vi "Measurement.vi"(0 "Position":T7(array[cluster]) {"Z" format="%.1f"; "Y" format="%.1f"; "X" format="%.1f"}, 1 "setup":T8=enum."Show Setup", 2 "Post Process":T5, 4 "File":T9, 5 "Results file":path, 7 "Raw data file":path, 11 "Setup filename":string) -> (14 "2nd plot":cluster{"Xo":dbl, "Delta X":dbl, dbl[]}[](graph), 19 "Status Out":T4)   [LabVIEW 2010]
uses:
  Anemometry Sub Vis/Controls/Save_Data.ctl
  Anemometry Sub Vis/Controls/Setup.ctl
  Anemometry Sub Vis/Controls/Graph_Type.ctl
  Anemometry Sub Vis/Controls/Post_Process.ctl
  Anemometry Sub Vis/Gen Trav/Multi_Run_Status.ctl
  Anemometry Sub Vis/Controls/Board_Types.ctl
  Anemometry Sub Vis/File/Setup_Filetype.ctl
  Anemometry Sub Vis/Controls/Block_start_and_end.ctl
  ADAM Client/Sub VIs/ADAM Controls/Traverse_Level_State.ctl
  Anemometry Sub Vis/Globals/Trav_pos_global.vi
  Anemometry Sub Vis/Globals/Meas_global.vi
  Anemometry Sub Vis/Acquisition/Data_Translation/DataTranslation_global.vi
  Anemometry Sub Vis/Acquisition/PWA/PWAtasksGLOBAL.vi
  Anemometry Sub Vis/Globals/Preference_global.vi
  Anemometry Sub Vis/Globals/LDA_meas_global_1.vi
  Anemometry Sub Vis/Globals/Dynamic_call_global.ph.vi
  Anemometry Sub Vis/Globals/LDA_meas_global_2.vi
  Anemometry Sub Vis/Globals/Plug_in_data_global.vi
panel:
  in  "PP next block":bool
  out "Pause message":string
  out "Statistics":string[][](table)
  in  "Tab Control":T1(tab)
  out "Measurement time (min)":dbl=6.0 format="%.2f"
  in  "No of bins":i32=80
  in  "Show Smoth":bool=TRUE
  in  "Second Graph":T3={"Plot 1"=2, "Plot 2"=1, "Save graph"=0, "Plot Type"=enum."Vel histogram"} {"Save graph" items=["Do not save plot", "Save plot"]; "Plot 2" items=["Nothing", "LDA (U)", "LDA (W)", "HW (HW) LDA Sync", "HW (HW)", "RV (WT)"]; "Plot 1" items=["Nothing", "LDA (U)", "LDA (W)", "HW (HW) LDA Sync", "HW (HW)", "RV (WT)"]}
  in  "First Graph":T3={"Plot 1"=1, "Plot 2"=2, "Save graph"=0, "Plot Type"=enum."Velocity trace"} {"Save graph" items=["Do not save plot", "Save plot"]; "Plot 2" items=["Nothing", "LDA (U)", "LDA (W)", "HW (HW) LDA Sync", "HW (HW)", "RV (WT)"]; "Plot 1" items=["Nothing", "LDA (U)", "LDA (W)", "HW (HW) LDA Sync", "HW (HW)", "RV (WT)"]}
  out "First plot":cluster{"Xo":dbl, "Delta X":dbl, dbl[]}[](graph)
  in  "Comments":string
  out "BSA Diagnostic info":string[][](table)
  out "uv":dbl[][](graph)=[[-0.041806189081711534, -0.046435429052714985, -0.04035660097427599, -0.042187605126076694, -0.042052555599004206]]
  out "u^4":dbl[][](graph)
  out "u^3":dbl[][](graph)
  out "u^2":dbl[][](graph)=[[0.09743628875280319, 0.10575821456272283, 0.10126262927293661, 0.09890442087602569, 0.1022948212436432]]
  out "U":dbl[][](graph)=[[0.8295029456391334, 0.8915896983798417, 0.8415763502225625, 0.8394746126219594, 0.8466062785395404]]
  in  "Block average display control":cluster{"Name":string, "Include":bool}[](array[cluster])=[{"Name"="FF (C)", "Include"=FALSE}]
  out "Array U":dbl[][](array[numeric]) format="%.2e"
  out "Array u^2":dbl[][](array[numeric]) format="%.2e"
  out "Actual Sampling freq":dbl=100.0 format="%.1f"
  in  "Desired Sampling freq (Hz)":dbl=100.0 format="%.1f"
  in  "Correlate?":T6(ring)
  out "Current Block No":i32=5
  in  "Pause":bool
  in  "No of Blocks":i32=5
  in  "stop":bool
  in  "No of samples":i32=1000 min=0 step=1
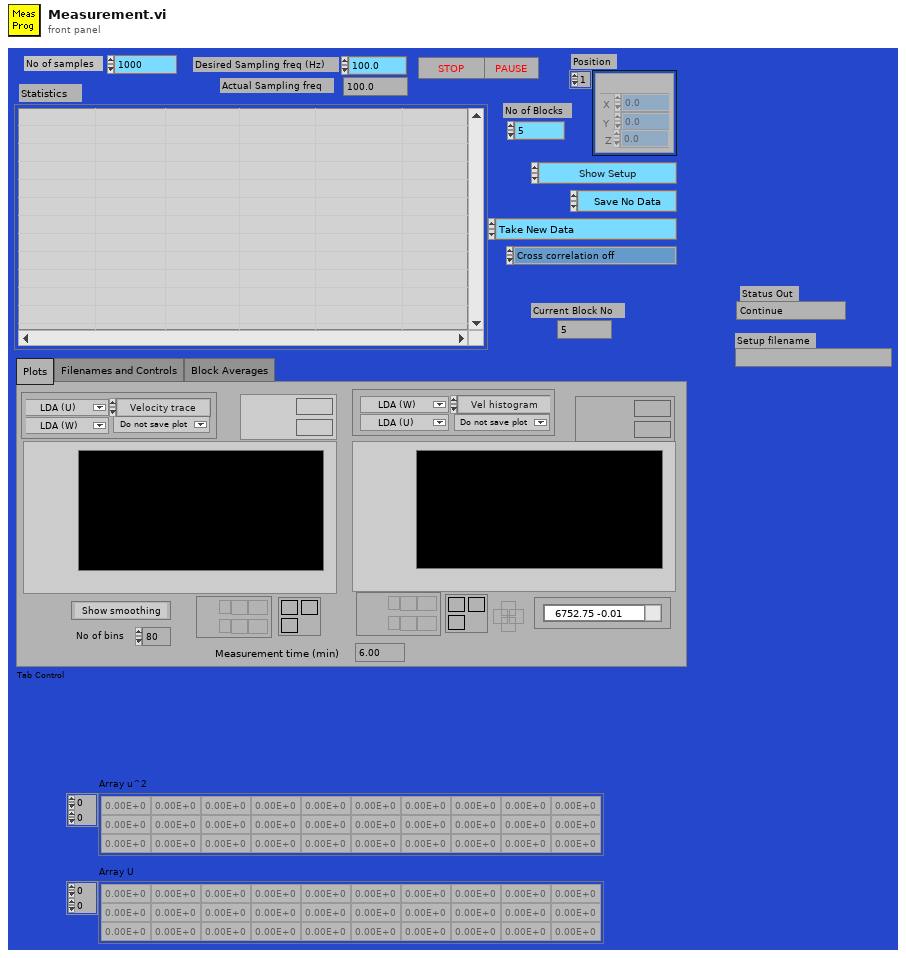
[diagram p1: front panel]
types:
  T1 = enum32{"Plots", "Filenames and Controls", "Block Averages"}
  T2 = typedef "Graph_Type.ctl" = enum16{"Show no graph", "Voltage trace", "Velocity trace", "Vel histogram", "Spectrum", "f.E(f) v Log f", "Auto-Corr"}
  T3 = cluster{"Plot 1":u16, "Plot 2":u16, "Save graph":u16, "Plot Type":T2}
  T4 = typedef "Multi_Run_Status.ctl" = enum16{"Continue", "Jump to Next Point", "Jump to Next Row", "Jump To Fall Back", "Terminate Run"}
  T5 = typedef "Post_Process.ctl" = enum16{"Take New Data", "Post Process Raw Data File"}
  T6 = enum16{"Cross correlation off", "Show correlation panel", "Correlate without activating panel"}
  T7 = cluster{"Name":string, "X":dbl, "Y":dbl, "Z":dbl}[]
  T8 = typedef "Setup.ctl" = enum16{"Run Program", "Show Setup", "Save Current Setup", "Setup Front Panel"}
  T9 = typedef "Save_Data.ctl" = enum16{"Save No Data", "Save Data"}
  T10 = enum32{"Bad", "Idle", "Run top level", "Running"}
  T11 = enum16{"Velocity", "Transit time", "Arrival time"}
  T12 = enum16{"Save no data", "Save data in new files", "Save data in existing files"}
  T13 = typedef "Board_Types.ctl" = enum16{"Simulate", "Local ADAM", "Server ADAM", "NI-DAQmx", "NI-DAQmxBase", "ADC488", "DT LV-link"}
  T14 = typedef "Setup_Filetype.ctl" = enum16{"Measurement Setups", "Calibration Setups", "General", "Results File Plotter Setups", "Speed Calib Tweaks"}
  T15 = typedef "Block_start_and_end.ctl" = cluster{"Started":dbl, "Ended":dbl, "Analogue Frequency Hz":dbl}
  T16 = typedef "Traverse_Level_State.ctl" = enum16{"Running", "Complete"}
  T17 = typedef "Traverse_cluster.ctl" = cluster{"Start X":dbl, "Start Y":dbl, "Start Z":dbl, "End X":dbl, "End Y":dbl, "End Z":dbl, "No. of pts.":i32, "Spacing":T18, "Filename":path, "Tunnel Speed":dbl, "Averaging time (min)":dbl, "Extra Commands":string, "Specific Arguments":string, "Emission Rate (l/min)":dbl, "Trace Gas Concentration (%)":dbl, "Density Ratio":string, "Comments":string, "Row No":i32, "Row Type Selector":T19, "Completion time":string, "Row Duration (mins)":dbl, "No. of Valid pts.":i32, "Meas Setup File":string}
  T18 = typedef "Spacing.ctl" = enum16{"Linear", "Log", "Gauss", "Specified", "N/A"}
  T19 = typedef "Multi_run_mode.ctl" = enum16{"Move Traverse Only", "Set Tunnel Speed Only", "Set Source Only", "Set Measurement Conditions", "Single Measurement", "Vertical Profile", "Lateral Profile", "Longitudinal Profile", "Explore Volume", "Multi-Axis Profile", "Auto Calibrate", "Meas Fast FID Bkgnd", "Check Beam Power", "Scanning Valve Measurement", "Run VI Named:", "Set ADAM Ch", "Wait (minutes)", "Send Message", "Synchronize With:", "Fall Back to this Row", "Turn Off Row Repeating", "Blank Row"}
  T20 = typedef "Analysis_info_cluster.ctl" = cluster{"Colour":u32, "Inst type":T21, "Inst name":string, "Symbol":string, "Code name":string, "Extra Info":string, "Inst Array":T22, "Index":i32, "Voltage Index":i32, "Extra Titles":string[], "Extra Values":string[]}
  T21 = typedef "Inst_type.ctl" = enum16{"Propeller anemometer", "Raw voltage", "Pressure Transducer", "Pitot-static tube", "Preston tube", "Hot wire", "Cross wire 1", "Cross wire 2", "Generic Linear", "Generic Polynomial", "Generic BackPoly", "Fast FID", "Thermocouple", "Cold wire", "Pulsed Wire", "LDA Vel", "LDA Tran time", "LDA Arr time"}
  T22 = typedef "Instrument_Array.ctl" = enum16{"PWA", "LDA", "Analogue"}
  T23 = enum16{"Velocity", "Transit time", "Arrival time"}[]
  T24 = typedef "BSA_Type.ctl" = enum16{"57N11", "BSA F60"}
  T25 = typedef "BSA_info_Cluster.ctl" = cluster{"GPIB Address":string, "No of Check Bytes":i32, "Extra Info":string, "COLOUR":u32, "Wavelength (nm)":dbl}
  T26 = typedef "Ch_and_Spans.ctl" = cluster{"high limit (10V)":sgl, "low limit (-10V)":sgl, "Ch No":i16, "Var name":string, "Use Latest Calib":bool}
  T27 = typedef "Velocity_cluster.ctl" = cluster{"Name":string, "U":dbl, "u^2":dbl, "u^3/(u^2)^(1.5)":dbl, "u^4/(u^2)^2 -3":dbl, "% u'/U":dbl, "Mean % Err":dbl, "u^4":dbl}
  T28 = typedef "Analysis_type_cluster.ctl" = cluster{"Analysis type":T29, "Indicies":i32[], "Name":string, "Inst Array":T22, "Info index":i32}
  T29 = typedef "Analysis_type_Enum.ctl" = enum16{"Slow Response", "Fast Response", "Weighted Fast Response", "Fast FID", "Weighted Fast FID", "Cross Wire", "Weighted Cross Wire", "Weighted LDA"}
  T30 = cluster{"Insts for plotting[0]":u16, "Insts for plotting[1]":u16}
  T31 = typedef "PWA_Data.ctl" = enum16{"No PWA Data", "One Ch PWA"}
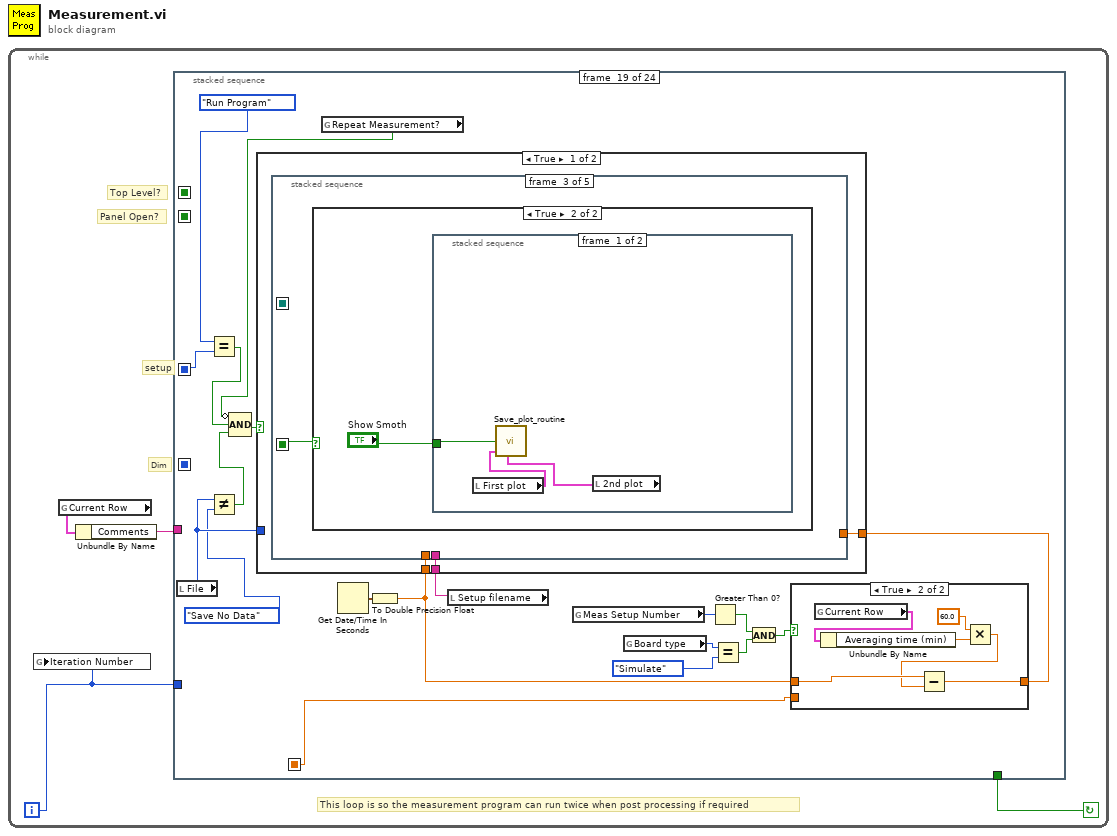
[diagram p0: block diagram]
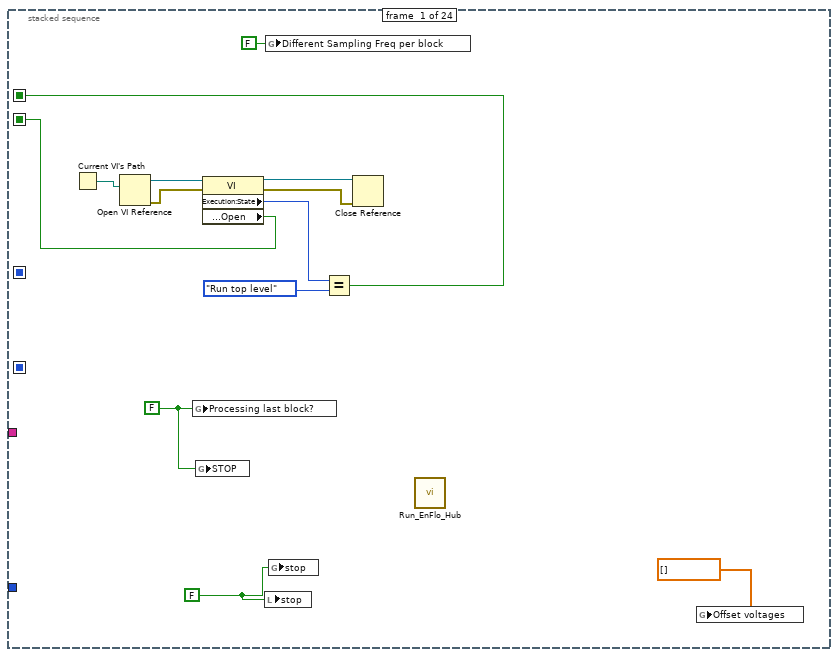
[diagram p2: hidden frame]
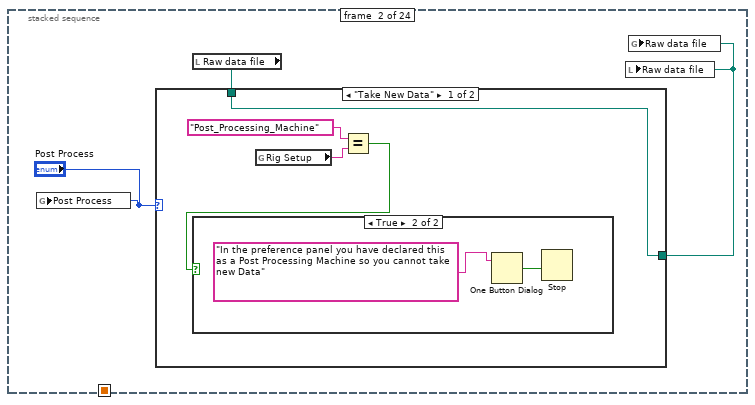
[diagram p3: hidden frame]
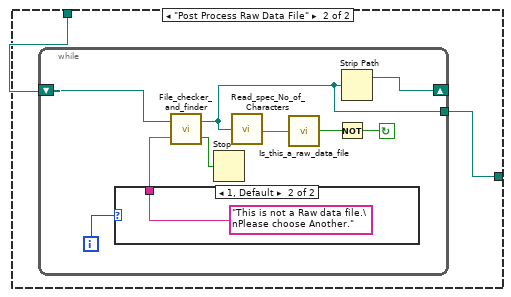
[diagram p5: hidden frame]
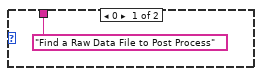
[diagram p6: hidden frame]
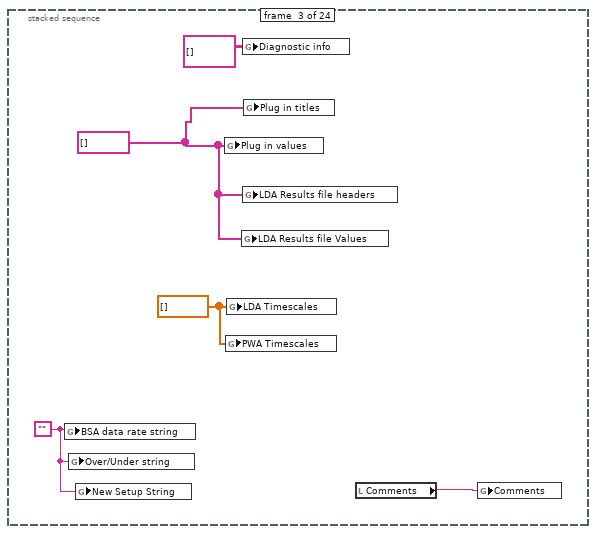
[diagram p7: hidden frame]
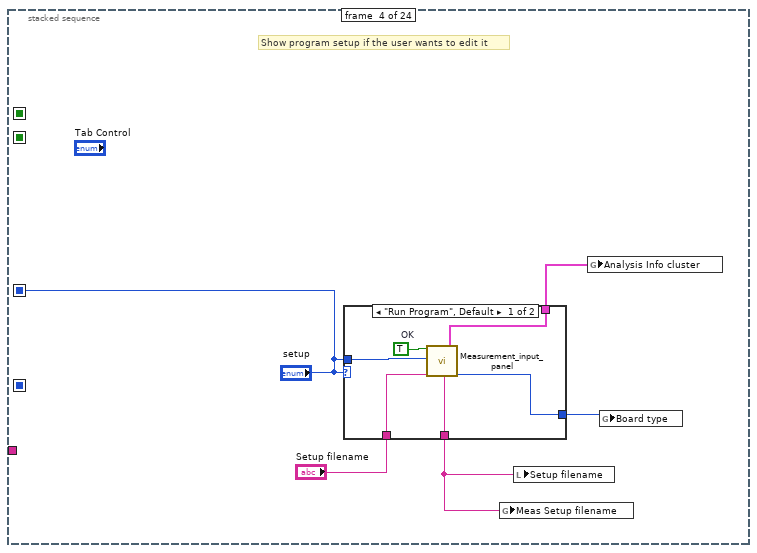
[diagram p8: hidden frame]
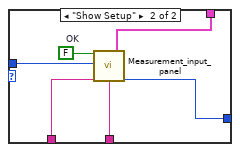
[diagram p9: hidden frame]
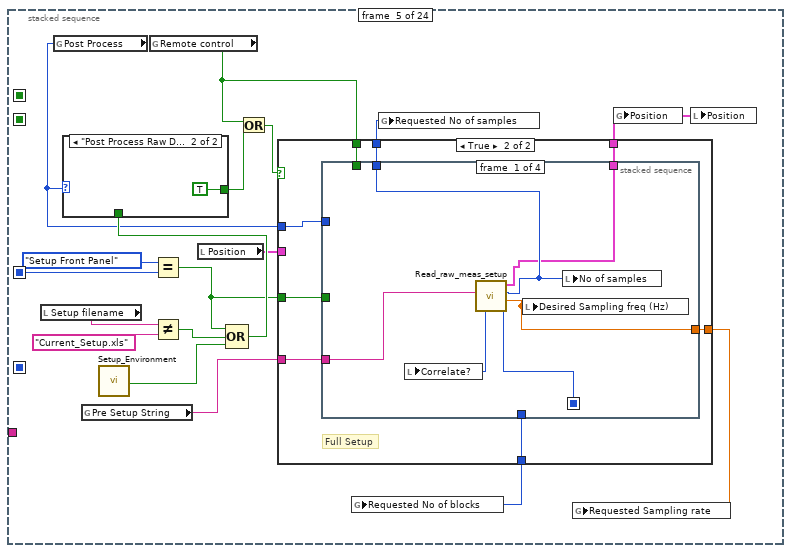
[diagram p10: hidden frame]
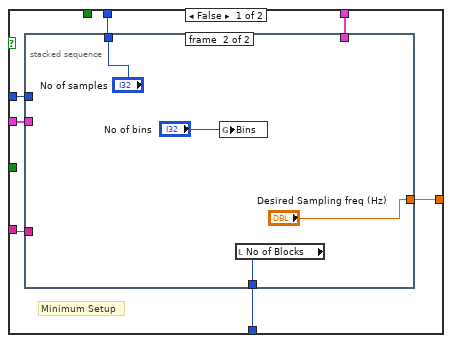
[diagram p12: hidden frame]
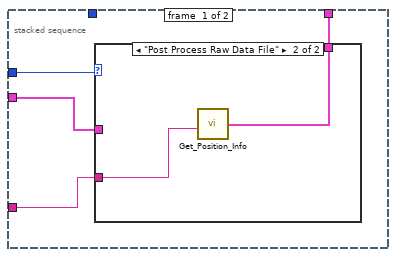
[diagram p13: hidden frame]
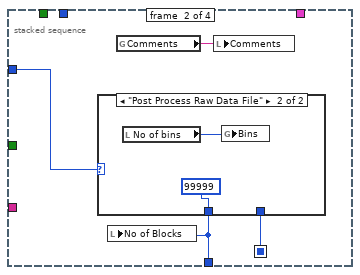
[diagram p15: hidden frame]
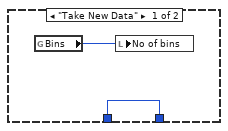
[diagram p16: hidden frame]
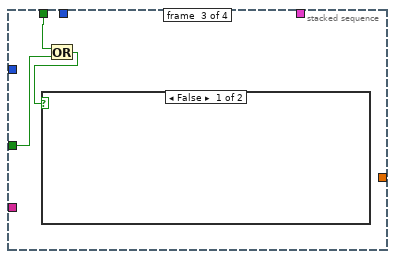
[diagram p17: hidden frame]
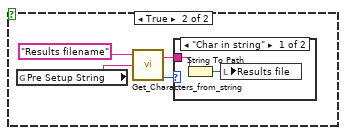
[diagram p18: hidden frame]
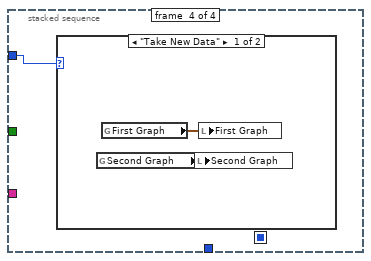
[diagram p20: hidden frame]
diagram:
  n1 = while {
    i -> [w1]
    stop <- w2 continue-if-true
    # "This loop is so the measurement program can run twice when post processing if required"
    # "Panel Open?"
    # "Top Level?"
    # "setup"
    # "Dim"
    n2 = global write "Meas_global.vi" "Iteration Number"(w1) -> ()
    n3 = global read "Trav_pos_global.vi" "Current Row"() -> (w3:T17)
    n4 = Unbundle By Name(w3) -> ("Comments"=w4:string)
    n5 = stacked-sequence {
      seq-local: [_ _ _ _ _ _ _ _ w187 _ _ _ _ _ _ _ _ _ _ _ _ _ _ _] -> [_ _ _ _ _ _ _ _ _ _ _ _ _ _ _ _ _ w625 _ _ _ _ _ _]
      seq-local: [_ _ _ "setup" _ _ _ _ _ _ _ _ _ _ _ _ _ _ _ _ _ _ _ _] -> [_ _ _ _ w71 _ _ _ w179 w264 _ _ _ _ w525 w563 w570 w626 w934 w1010 w1038 _ _ w1115]
      seq-local: [_ _ _ _ _ _ _ _ _ _ _ _ _ _ _ _ w566 _ _ _ _ _ _ _] -> [_ _ _ _ _ _ _ _ _ _ _ _ _ _ _ _ _ w624 w917 _ _ _ _ _]
      seq-local: [w7 _ _ _ _ _ _ _ _ _ _ _ _ _ _ _ _ _ _ _ _ _ _ _] -> [_ _ _ _ _ _ _ _ _ w244 _ _ _ _ w521 _ _ w623 _ _ _ _ _ _]
      seq-local: [w6 _ _ _ _ _ _ _ _ _ _ _ _ _ _ _ _ _ _ _ _ _ _ _] -> [_ _ _ _ _ _ _ _ _ _ _ _ w364 _ _ _ _ _ _ _ _ _ _ _]
      tunnel: w4 -> [_ _ _ _ _ _ _ w172 _ _ _ _ _ _ _ _ _ _ _ _ _ _ w1081 _]
      tunnel: w1 -> [_ _ _ _ _ _ _ _ _ _ _ _ _ _ _ _ _ _ _ _ _ _ w1076 _]
      tunnel: [_ _ _ _ _ _ _ _ _ _ _ _ _ _ _ _ _ _ _ _ _ _ w1075 _] -> w2
      frame #0 {
        w15 = FALSE ("Processing last block?")
        w16 = FALSE ("stop")
        n6 = Current VI's Path() -> (path=w8:path)
        n7 = Open VI Reference(vi path=w8) -> (vi reference=w9:refnum<vi>, error out=w10:errorcluster)  [unwired: 1 in, 4 out]
        n8 = global write "Meas_global.vi" "Processing last block?"(w15) -> ()
        n9 = global write "PWAtasksGLOBAL.vi" "STOP"(w15) -> ()
        n10 = property class="VI"(reference=w9, error in=w10) -> (reference out=w11:refnum<vi>, error out=w12:errorcluster, "Execution:State"=w13:T10, "Front Panel.Open"=w6:bool)
        n11 = local write "stop"(w16) -> ()
        n12 = global write "DataTranslation_global.vi" "Different Sampling Freq per block"(FALSE ("Different Sampling Freq per block")) -> ()
        n13 = global write "Meas_global.vi" "stop"(w16) -> ()
        n14 = Equal?(x=w13, y=T10."Run top level" ("Exec.State")) -> (x = y?=w7:bool)
        n15 = Close Reference(reference=w11, error in (no error)=w12) -> ()  [unwired: 1 out]
        n16 = call "Run_EnFlo_Hub.vi"() -> ()  [unwired: 8 out]
        n17 = global write "Meas_global.vi" "Offset voltages"(dbl[] [] ("Offset voltages used")) -> ()
      }
      frame #1 {
        n18 = global write "Meas_global.vi" "Post Process"("Post Process") -> ()
        n19 = local read "Raw data file"() -> (w20:path)
        n20 = case shown="\"Take New Data\"" "Post Process" {
          tunnel: [w24 w28] -> w19
          tunnel: w20 -> [w24 w27]
          frame "Take New Data" {
            n21 = global read "Preference_global.vi" "Rig Setup"() -> (w23:string)
            n22 = Equal?(x="Post_Processing_Machine" ("Rig Setup"), y=w23) -> (x = y?=w21:bool)
            n23 = case shown="True" w21 {
              frame False {
              }
              frame True {
                n24 = One Button Dialog(message="In the preference panel you have declared this as a Post Processing Machine so you cannot take new Data") -> (true=w25:bool)  [unwired: 1 in]
                n25 = Stop(stop? (T)=w25) -> ()
              }
            }
          }
          frame "Post Process Raw Data File" {
            n26 = while {
              tunnel: [w30] -> w28
              shift-left: w27 -> [w32]
              shift-right: [w31] -> _
              i -> [w33]
              stop <- w34 continue-if-true
              n27 = case shown="1, Default" w33 {
                tunnel: ["Find a Raw Data File to Post Process" ("Promp if not found") "This is not a Raw data file.\nPlease choose Another." ("Promp if not found")] -> w37
                frame 0 {
                }
                frame 1, Default {
                }
              }
              n28 = call "File_checker_and_finder.vi"("Promp if not found"=w37, "Filename In"=w32) -> ("cancelled"=w29:bool, "Filename Out"=w30:path)
              n29 = Stop(stop? (T)=w29) -> ()
              n30 = call "Read_spec_No_of_Characters.vi"("Filename"=w30) -> ("character string"=w36:string)  [unwired: 1 out]
              n31 = call "Is_this_a_raw_data_file.vi"("character string"=w36) -> ("Raw Dat File?"=w35:bool)  [unwired: 2 out]
              n32 = Not(x=w35) -> (.not. x?=w34:bool)
              n33 = Strip Path(path=w30) -> (stripped path=w31:path)  [unwired: 1 out]
            }
          }
        }
        n34 = local write "Raw data file"(w19) -> ()
        n35 = global write "Meas_global.vi" "Raw data file"(w19) -> ()
      }
      frame #2 {
        w42 = dbl[] [] ("LDA Timescales")
        w41 = string[] [] ("Plug in values")
        w44 = ""
        n36 = global write "Meas_global.vi" "BSA data rate string"(w44) -> ()
        n37 = global write "Meas_global.vi" "Over/Under string"(w44) -> ()
        n38 = global write "Meas_global.vi" "New Setup String"(w44) -> ()
        n39 = global write "Dynamic_call_global.ph.vi" "Plug in values"(w41) -> ()
        n40 = global write "PWAtasksGLOBAL.vi" "PWA Timescales"(w42) -> ()
        n41 = global write "LDA_meas_global_1.vi" "LDA Timescales"(w42) -> ()
        n42 = global write "LDA_meas_global_1.vi" "LDA Results file Values"(w41) -> ()
        n43 = global write "Meas_global.vi" "Diagnostic info"(string[][] [] ("Diagnostic info")) -> ()
        n44 = global write "LDA_meas_global_1.vi" "LDA Results file headers"(w41) -> ()
        n45 = global write "Dynamic_call_global.ph.vi" "Plug in titles"(w41) -> ()
        n46 = local read "Comments"() -> (w43:string)
        n47 = global write "Meas_global.vi" "Comments"(w43) -> ()
      }
      frame #3 {
        # "Show program setup if the user wants to edit it"
        n48 = case shown="\"Run Program\", Default" "setup" {
          tunnel: [w54 w60] -> w49
          tunnel: [w53 w59] -> w48
          tunnel: "Setup filename" -> [w52 w58]
          tunnel: [w51 w57] -> w45
          tunnel: "setup" -> [w50 w56]
          frame "Run Program", Default {
            w55 = TRUE  # OK
            n49 = call "Measurement_input_panel.vi"("OK"=w55, "setup"=w50, "Setup filename"=w52) -> ("Setup filename out"=w51:string, "Analysis Info cluster"=w54:T20[], "Board type"=w53:T13)  [unwired: 14 out]
          }
          frame "Show Setup" {
            w61 = FALSE  # OK
            n50 = call "Measurement_input_panel.vi"("OK"=w61, "setup"=w56, "Setup filename"=w58) -> ("Setup filename out"=w57:string, "Analysis Info cluster"=w60:T20[], "Board type"=w59:T13)  [unwired: 14 out]
          }
        }
        n51 = global write "Meas_global.vi" "Meas Setup filename"(w45) -> ()
        n52 = local write "Setup filename"(w45) -> ()
        n53 = global write "Meas_global.vi" "Analysis Info cluster"(w49) -> ()
        n54 = global write "Meas_global.vi" "Board type"(w48) -> ()
      }
      frame #4 {
        n55 = local read "Setup filename"() -> (w75:string)
        n56 = global read "Meas_global.vi" "Post Process"() -> (w70:T5)
        n57 = global read "Meas_global.vi" "Pre Setup String"() -> (w66:string)
        n58 = call "Setup_Environment.vi"() -> ("First Time"=w67:bool)  [unwired: 1 in]
        n59 = global read "Meas_global.vi" "Remote control"() -> (w63:bool)
        n60 = Equal?(x=Setup."Setup Front Panel" ("setup"), y=w71) -> (x = y?=w62:bool)
        n61 = Not Equal?(x=w75, y="Current_Setup.xls" ("Setup filename")) -> (x != y?=w73:bool)
        n62 = local read "Position"() -> (w64:T7)
        n63 = Compound Arithmetic op=OR(w62, w73, w67) -> (w72:bool)
        n64 = case shown="\"Post Process Raw Data File\"" w70 {
          tunnel: [w80 TRUE] -> w79
          tunnel: w72 -> [w80 _]
          frame "Take New Data" {
          }
          frame "Post Process Raw Data File" {
          }
        }
        n65 = Or(x=w63, y=w79) -> (x .or. y?=w78:bool)
        n66 = case shown="True" w78 {
          tunnel: w70 -> [w84 w107]
          tunnel: [w88 w106] -> w68
          tunnel: [w87 w101] -> w77
          tunnel: [w86 w105] -> w76
          tunnel: [w85 w104] -> w65
          tunnel: w66 -> [w83 w103]
          tunnel: w64 -> [w82 _]
          tunnel: w63 -> [_ w102]
          tunnel: w62 -> [_ w100]
          frame False {
            # "Minimum Setup"
            n67 = stacked-sequence {
              tunnel: [_ "Desired Sampling freq (Hz)"] -> w88
              tunnel: [_ w98] -> w87
              tunnel: [_ "No of samples"] -> w86
              tunnel: [w91 _] -> w85
              tunnel: w84 -> [w92 _]
              tunnel: w83 -> [w90 _]
              tunnel: w82 -> [w89 _]
              frame #0 {
                n68 = case shown="\"Post Process Raw Data File\"" w92 {
                  tunnel: [w93 w94] -> w91
                  tunnel: w89 -> [w93 _]
                  tunnel: w90 -> [_ w95]
                  frame "Take New Data" {
                  }
                  frame "Post Process Raw Data File" {
                    n69 = call "Get_Position_Info.vi"("Input string"=w95) -> ("Position"=w94:T7)
                  }
                }
              }
              frame #1 {
                n70 = global write "Meas_global.vi" "Bins"("No of bins") -> ()
                n71 = local read "No of Blocks"() -> (w98:i32)
              }
            }
          }
          frame True {
            # "Full Setup"
            n72 = stacked-sequence {
              seq-local: [w110 _ _ _] -> [_ w115 _ _]
              tunnel: w107 -> [_ w116 _ w131]
              tunnel: [w113 _ _ _] -> w106
              tunnel: [w112 _ _ _] -> w105
              tunnel: [w108 _ _ _] -> w104
              tunnel: w103 -> [w111 _ _ _]
              tunnel: w102 -> [_ _ w124 _]
              tunnel: [_ w114 _ _] -> w101
              tunnel: w100 -> [_ _ w123 _]
              frame #0 {
                n73 = call "Read_raw_meas_setup.vi"("Setup file string"=w111) -> ("No of Blocks"=w110:i32, "Sampling freq (Hz)"=w113:dbl, "No of samples"=w112:i32, "Position"=w108:T7, "Correlate?"=w109:T6)  [unwired: 4 out]
                n74 = local write "Correlate?"(w109) -> ()
                n75 = local write "Desired Sampling freq (Hz)"(w113) -> ()
                n76 = local write "No of samples"(w112) -> ()
              }
              frame #1 {
                n77 = case shown="\"Post Process Raw Data File\"" w116 {
                  tunnel: [w119 99999 ("No of Blocks")] -> w114
                  tunnel: w115 -> [w119 _]
                  frame "Take New Data" {
                    n78 = global read "Meas_global.vi" "Bins"() -> (w118:i32)
                    n79 = local write "No of bins"(w118) -> ()
                  }
                  frame "Post Process Raw Data File" {
                    n80 = local read "No of bins"() -> (w120:i32)
                    n81 = global write "Meas_global.vi" "Bins"(w120) -> ()
                  }
                }
                n82 = local write "No of Blocks"(w114) -> ()
                n83 = global read "Meas_global.vi" "Comments"() -> (w117:string)
                n84 = local write "Comments"(w117) -> ()
              }
              frame #2 {
                n85 = Or(x=w124, y=w123) -> (x .or. y?=w122:bool)
                n86 = case shown="False" w122 {
                  frame False {
                  }
                  frame True {
                    n87 = global read "Meas_global.vi" "Pre Setup String"() -> (w125:string)
                    n88 = call "Get_Characters_from_string.vi"("Input string"=w125, "Variable name"="Results filename") -> ("Status"=w128:enum16{"Char in string", "Char not in string"}, "Value"=w127:string)  [unwired: 1 in]
                    n89 = case shown="\"Char in string\"" w128 {
                      tunnel: w127 -> [w130 _]
                      frame "Char in string" {
                        n90 = String To Path(string=w130) -> (path=w129:path)
                        n91 = local write "Results file"(w129) -> ()
                      }
                      frame "Char not in string" {
                      }
                    }
                  }
                }
              }
              frame #3 {
                n92 = case shown="\"Take New Data\"" w131 {
                  frame "Take New Data" {
                    n93 = global read "Meas_global.vi" "Second Graph"() -> (w132:T3)
                    n94 = global read "Meas_global.vi" "First Graph"() -> (w133:T3)
                    n95 = local write "Second Graph"(w132) -> ()
                    n96 = local write "First Graph"(w133) -> ()
                  }
                  frame "Post Process Raw Data File" {
                  }
                }
              }
            }
          }
        }
        n97 = global write "Meas_global.vi" "Requested No of blocks"(w77) -> ()
        n98 = global write "Meas_global.vi" "Requested No of samples"(w76) -> ()
        n99 = global write "Meas_global.vi" "Requested Sampling rate"(w68) -> ()
        n100 = global write "Meas_global.vi" "Position"(w65) -> ()
        n101 = local write "Position"(w65) -> ()
      }
      frame #5 {
        n102 = global read "Meas_global.vi" "Post Process"() -> (w134:T5)
        n103 = case shown="\"Post Process Raw Data File\"" w134 {
          tunnel: [w137 w138] -> w135
          frame "Take New Data" {
            n104 = Get Date/Time In Seconds() -> (seconds since 1Jan1904=w136:timestamp)
            n105 = To Double Precision Float(number=w136) -> (double precision float=w137:dbl)
          }
          frame "Post Process Raw Data File" {
            n106 = global read "Meas_global.vi" "Pre Setup String"() -> (w141:string)
            n107 = call "Get_Characters_from_string.vi"("Input string"=w141, "Variable name"="Seconds since 1/1/04") -> ("Value"=w139:string)  [unwired: 1 in, 1 out]
            n108 = call "String_2_Number.vi"("Value"=w139) -> ("Numeric"=w138:dbl)
          }
        }
        n109 = global write "Meas_global.vi" "Time Data was Aquired"(w135) -> ()
      }
      frame #6 {
        n110 = global read "Dynamic_call_global.ph.vi" "Initial Plug Ins"() -> (w143:string[])
        n111 = global read "Dynamic_call_global.ph.vi" "Initial Plug Ins Extra"() -> (w144:string[])
        n112 = Build Array (concatenate)(w144, w143) -> (w142:string[])
        n113 = Array Size(array=w142) -> (size(s)=w146:i32)
        n114 = Greater Than 0?(x=w146) -> (x > 0?=w145:bool)
        n115 = case shown="True" w145 {
          tunnel: w142 -> [_ w147]
          frame False {
          }
          frame True {
            n116 = stacked-sequence {
              tunnel: w147 -> [w149 _]
              frame #0 {
                n117 = global read "Meas_global.vi" "Post Process"() -> (w151:T5)
                n118 = call "Plug_in_Directories.vi"() -> ("Initial"=w148:path)  [unwired: 3 out]
                n119 = Equal?(x=w151, y=Post_Process."Post Process Raw Data File" ("Post Process")) -> (x = y?=w150:bool)
                n120 = for {
                  tunnel: w150 -> [w157]
                  tunnel: w149 -> [w154] mode=indexing
                  tunnel: w148 -> [w153]
                  w164 = FALSE  # Dialog Box (T)
                  n121 = Build Path(base path=w153, name or relative path=w154) -> (appended path=w155:path)
                  n122 = Open VI Reference(vi path=w155) -> (vi reference=w162:refnum<vi>, error out=w161:errorcluster)  [unwired: 2 in, 3 out]
                  n123 = property class="VI"(reference=w162, error in=w161, "Front Panel Window:Open"=TRUE ("Wait until done")) -> (reference out=w160:refnum<vi>, error out=w159:errorcluster)
                  n124 = invoke class="VI" method="Run VI"(reference=w160, error in=w159, "Wait until done"=w157, "Auto Dispose Ref"=FALSE) -> (reference out=w167:refnum<vi>, error out=w166:errorcluster)  [unwired: 1 in, 3 out]
                  n125 = Close Reference(reference=w167, error in (no error)=w166) -> (error out=w165:errorcluster)
                  n126 = call "EnFlo_Error_Handler.vi"("error in (no error)"=w165, "Error Type"="Launching Initial Plug In", "Dialog Box (T)"=w164) -> ()  [unwired: 3 out]
                }
              }
              frame #1 {
                n127 = global read "Meas_global.vi" "Requested No of blocks"() -> (w169:i32)
                n128 = global read "Meas_global.vi" "Comments"() -> (w168:string)
                n129 = local write "Comments"(w168) -> ()
                n130 = local write "No of Blocks"(w169) -> ()
              }
            }
          }
        }
      }
      frame #7 {
        n131 = local read "Comments"() -> (w173:string)
        n132 = Concatenate Strings(w172, w173) -> (w171:string)
        n133 = call "Text_without_format.vi"("Input string"=w171) -> ("Output string"=w170:string)
        n134 = local write "Comments"(w170) -> ()
        n135 = global write "Meas_global.vi" "Comments"(w170) -> ()
      }
      frame #8 {
        n136 = global read "Meas_global.vi" "dimensions"() -> (w187:enum16{"1D", "2D"})
        n137 = global read "Meas_global.vi" "Post Process"() -> (w186:T5)
        n138 = global read "Meas_global.vi" "LDA data"() -> (w184:enum16{"No LDA data", "Take LDA data"})
        n139 = Equal?(x=Setup."Run Program" ("setup"), y=w179) -> (x = y?=w182:bool)
        n140 = Equal?(x=w179, y=Setup."Show Setup" ("setup")) -> (x = y?=w174:bool)
        n141 = Equal?(x=w184, y=enum16{"No LDA data", "Take LDA data"}."Take LDA data" ("LDA data")) -> (x = y?=w177:bool)
        n142 = Or(x=w182, y=w174) -> (x .or. y?=w176:bool)
        n143 = Equal?(x=w186, y=Post_Process."Take New Data" ("Post Process")) -> (x = y?=w178:bool)
        n144 = Compound Arithmetic op=AND(w176, w177, w178) -> (w175:bool)
        n145 = case shown="True" w175 {
          tunnel: w187 -> [_ w196]
          tunnel: w179 -> [_ w195]
          tunnel: w174 -> [_ w193]
          frame False {
            n146 = global write "LDA_meas_global_1.vi" "Number of measured quantities"(3 ("Number of measured quantities")) -> ()
            n147 = Build Array(T11."Velocity", T11."Transit time", T11."Arrival time") -> (w188:T23)
            n148 = global write "LDA_meas_global_2.vi" "data type"(w188) -> ()
            n149 = global write "LDA_meas_global_1.vi" "data type"(w188) -> ()
          }
          frame True {
            n150 = global read "LDA_meas_global_1.vi" "BSA Type"() -> (w194:T24)
            n151 = case shown="\"BSA F60\"" w194 {
              tunnel: w196 -> [w198 _]
              tunnel: w195 -> [w197 _]
              tunnel: w193 -> [_ w234]
              frame "57N11" {
                n152 = stacked-sequence {
                  tunnel: w198 -> [w201 w227]
                  tunnel: w197 -> [w200 _]
                  frame #0 {
                    n153 = global read "Meas_global.vi" "Remote control"() -> (w199:bool)
                    n154 = case shown="\"2D\"" w201 {
                      tunnel: w200 -> [w203 w216]
                      tunnel: w199 -> [w202 w215]
                      frame "2D" {
                        n155 = while {
                          tunnel: w202 -> [w204]
                          tunnel: w203 -> [w205]
                          stop <- w206 continue-if-true
                          n156 = stacked-sequence {
                            tunnel: [_ _ w212] -> w206
                            tunnel: w205 -> [w207 w209 _]
                            tunnel: w204 -> [_ _ w211]
                            frame #0 {
                              w208 = "1"  # BSA Number
                              n157 = call "Control_BSA_setup.vi"("setup"=w207, "BSA number"=w208) -> ()  [unwired: 14 out]
                            }
                            frame #1 {
                              w210 = "2"  # BSA Number
                              n158 = call "Control_BSA_setup.vi"("setup"=w209, "BSA number"=w210) -> ()  [unwired: 14 out]
                            }
                            frame #2 {
                              n159 = case shown="False" w211 {
                                tunnel: [w213 FALSE ("ok")] -> w212
                                frame False {
                                n160 = call "BSA_setup_check.vi"() -> ("ok"=w213:bool)
                                }
                                frame True {
                                }
                              }
                            }
                          }
                        }
                      }
                      frame "1D" {
                        n161 = stacked-sequence {
                          tunnel: w216 -> [w217 _]
                          tunnel: w215 -> [_ _]
                          frame #0 {
                            w218 = "1"  # BSA Number
                            n162 = call "Control_BSA_setup.vi"("setup"=w217, "BSA number"=w218) -> ()  [unwired: 14 out]
                          }
                          frame #1 {
                            n163 = global read "LDA_meas_global_2.vi" "BSA2 info"() -> (w219:T25)
                            n164 = Unbundle By Name(w219) -> ("GPIB Address"=w220:string)
                            n165 = call "Set_BSA_Coincidence.vi"("GPIB address"=w220, "Set Coincidence"=enum16{"Slave", "Master", "Private"}."Slave") -> ()  [unwired: 1 in, 5 out]
                          }
                        }
                      }
                    }
                  }
                  frame #1 {
                    n166 = global read "Meas_global.vi" "Remote control"() -> (w225:bool)
                    n167 = Equal?(x=w227, y=enum16{"1D", "2D"}."2D" ("dimensions")) -> (x = y?=w223:bool)
                    n168 = Not(x=w225) -> (.not. x?=w224:bool)
                    n169 = And(x=w224, y=w223) -> (x .and. y?=w222:bool)
                    n170 = case shown="True" w222 {
                      frame False {
                      }
                      frame True {
                        n171 = global read "LDA_meas_global_1.vi" "BSA1 info"() -> (w229:T25)
                        n172 = global read "LDA_meas_global_2.vi" "BSA2 info"() -> (w230:T25)
                        n173 = Build Array(w229, w230) -> (w228:T25[])
                        n174 = for {
                          tunnel: w228 -> [w232] mode=indexing
                          n175 = Unbundle By Name(w232) -> ("GPIB Address"=w231:string)
                          n176 = call "Set_BSA_Coincidence.vi"("GPIB address"=w231, "Set Coincidence"=enum16{"Slave", "Master", "Private"}."Master") -> ()  [unwired: 1 in, 5 out]
                        }
                      }
                    }
                  }
                }
              }
              frame "BSA F60" {
                n177 = disable-structure shown="TARGET_TYPE==Windows" {
                  disable-tunnel: w234 -> [_ w235]
                  frame condition #0 (active) {
                  }
                  frame condition #1 {
                    n178 = while {
                      tunnel: w235 -> [w238]
                      stop <- w236 continue-if-true
                      n179 = call "Edit_BSA_IP.vi"("Show Panel"=w238) -> ("Run LDA Diagnostic Out"=w237:bool)  [unwired: 2 out]
                      n180 = case shown="False" w237 {
                        tunnel: [FALSE w240] -> w236
                        frame False {
                        }
                        frame True {
                          n181 = call "F60_Diagnostic.vi"() -> ("Edit BSA Setup Out"=w240:bool)  [unwired: 11 in]
                        }
                      }
                    }
                  }
                }
              }
            }
          }
        }
      }
      frame #9 {
        w249 = Save_Data."Save No Data" ("File")
        w265 = Post_Process."Take New Data"  # Post Process
        n182 = global read "Trav_pos_global.vi" "Meas Setup Number"() -> (w245:i32)
        n183 = Not Equal?(x=Setup."Run Program" ("setup"), y=w264) -> (x != y?=w250:bool)
        n184 = call "Current_Filepath.vi"("Filename in"="Results file", "Data Type"="Results") -> ("Filename Out"=w243:path)  [unwired: 1 out]
        n185 = global read "Meas_global.vi" "Remote control"() -> (w261:bool)
        n186 = global read "Meas_global.vi" "Post Process"() -> (w252:T5)
        n187 = Equal?(x="File", y=w249) -> (x = y?=w259:bool)
        n188 = case shown="1, Default" w245 {
          tunnel: [w268 w270] -> w246
          tunnel: w243 -> [w268 w277]
          tunnel: w245 -> [_ w278]
          frame 0 {
          }
          frame 1, Default {
            n189 = Add(x=96, y=w278) -> (x+y=w280:i32)
            n190 = Build Array(w280) -> (w281:i32[])
            n191 = Strip Path(path=w277) -> (stripped path=w271:path, name=w276:string)
            n192 = Byte Array To String(unsigned byte array=w281) -> (string=w274:string)
            n193 = call "Add_filename_suffix.vi"("Filename"=w276) -> ("Original Suffix"=w273:string, "Base name"=w275:string)  [unwired: 1 in, 2 out]
            n194 = Format Into String(format string="%s_%s%s", w275, w274, w273) -> (resulting string=w272:string)  [unwired: 2 in, 1 out]
            n195 = Build Path(base path=w271, name or relative path=w272) -> (appended path=w270:path)
          }
        }
        n196 = Equal?(x=w252, y=w265) -> (x = y?=w251:bool)
        n197 = And(x=w261, y=w251) -> (x .and. y?=w257:bool)
        n198 = Compound Arithmetic op=AND(w259, invert w261, w251, invert w250) -> (w260:bool)
        n199 = while {
          shift-left: _ -> [w286]
          shift-right: [w283] -> _
          tunnel: "File" -> [w284]
          tunnel: [w287] -> w258
          tunnel: w260 -> [w283]
          stop <- FALSE continue-if-true
          n200 = Compound Arithmetic op=AND(w283, invert w286) -> (w285:bool)
          n201 = case shown="True" w285 {
            tunnel: [w288 w291] -> w287
            tunnel: w284 -> [w288 _]
            frame False {
            }
            frame True {
              n202 = Two Button Dialog(message="Do you wish to save the data?", 1:"Save Data" ("F button name (\"Cancel\")"), 2:"Save No Data" ("T button name (\"OK\")")) -> (T button?=w292:bool)
              n203 = Select(t=Save_Data."Save No Data" ("File"), s=w292, f=Save_Data."Save Data" ("File")) -> (s? t:f=w291:T9)
            }
          }
        }
        n204 = Equal?(x=w249, y=w258) -> (x = y?=w248:bool)
        n205 = Or(x=w248, y=w250) -> (x .or. y?=w263:bool)
        n206 = case shown="False" w263 {
          tunnel: w246 -> [w308 w316]
          tunnel: [w307 w316] -> w266
          tunnel: "Raw data file" -> [w306 w317]
          tunnel: [w301 w317] -> w255
          tunnel: w264 -> [w305 _]
          tunnel: w258 -> [w304 _]
          tunnel: [w302 T12."Save no data" ("File output")] -> w253
          tunnel: [w303 w314] -> w247
          tunnel: w257 -> [_ w311]
          tunnel: w250 -> [_ w310]
          tunnel: w244 -> [w300 _]
          frame False {
            n207 = call "File_setup.vi"("Measurement is top level?"=w300, "Results file"=w308, "Raw data file"=w306, "setup"=w305, "File"=w304) -> ("Results file output"=w307:path, "Raw data file output"=w301:path, "Raw data option"=w303:enum16{"Save raw data", "Raw data not saved"}, "File output"=w302:T12)
          }
          frame True {
            w312 = enum16{"Save raw data", "Raw data not saved"}."Raw data not saved"  # Raw data option
            n208 = global read "Meas_global.vi" "Raw data option"() -> (w313:enum16{"Save raw data", "Raw data not saved"})
            n209 = Compound Arithmetic op=AND(w311, invert w310) -> (w309:bool)
            n210 = Select(t=w313, s=w309, f=w312) -> (s? t:f=w314:enum16{"Save raw data", "Raw data not saved"})
          }
        }
        n211 = case shown="\"Save raw data\"" w247 {
          tunnel: w255 -> [w297 w299]
          tunnel: [w297 w298] -> w254
          frame "Raw data not saved" {
          }
          frame "Save raw data" {
            n212 = call "Find_Unique_Filename.vi"("Path In"=w299) -> ("Unique Path Out"=w298:path)  [unwired: 1 in, 1 out]
          }
        }
        n213 = case shown="\"Save data in new files\", Default" w253 {
          tunnel: w266 -> [_ w296]
          frame "Save no data" {
          }
          frame "Save data in new files", Default {
            n214 = local write "Results file"(w296) -> ()
            n215 = global write "Meas_global.vi" "Results file"(w296) -> ()
          }
        }
        n216 = global write "Meas_global.vi" "Raw data option"(w247) -> ()
        n217 = global write "Meas_global.vi" "File"(w253) -> ()
        n218 = global write "Meas_global.vi" "Raw data file"(w254) -> ()
        n219 = local write "Raw data file"(w254) -> ()
        n220 = local write "File"(w258) -> ()
      }
      frame #10 {
        n221 = global read "Meas_global.vi" "Ch & spans"() -> (w318:T26[])
        n222 = local read "Block average display control"() -> (w323:cluster{"Name":string, "Include":bool}[])
        n223 = global read "Meas_global.vi" "Velocity Cluster Array"() -> (w322:T27[])
        n224 = global write "Meas_global.vi" "Ch & spans + mod limits"(w318) -> ()
        n225 = global read "Meas_global.vi" "Analysis Info cluster"() -> (w328:T20[])
        n226 = call "Determine_Meas_Analysis.vi"("Analogue Channels"=w328) -> ("Analysis Info Cluster"=w325:T20[], "Analysis Type Array"=w327:T28[])
        n227 = for {
          tunnel: w325 -> [w338] mode=indexing
          tunnel: w323 -> [w337]
          tunnel: w322 -> [w335]
          tunnel: [w329] -> w321 mode=indexing
          tunnel: [w332] -> w320 mode=indexing
          tunnel: [w331] -> w319 mode=indexing
          i -> [w336]
          w330 = nan ("Mean % Err")
          n228 = Unbundle By Name(w338) -> ("Inst name"=w329:string)
          n229 = Index Array(array=w335, index=w336) -> (element=w334:T27)
          n230 = Index Array(array=w337, index=w336) -> (element=w333:cluster{"Name":string, "Include":bool})
          n231 = Bundle By Name(cluster=w333, "Name"=w329) -> (w332:cluster{"Name":string, "Include":bool})
          n232 = Bundle By Name(cluster=w334, "Name"=w329, "Mean % Err"=w330, "% u'/U"=w330) -> (w331:T27)
        }
        n233 = Build Array (concatenate)("Nothing", w321) -> (w324:string[])
        n234 = local write "Block average display control"(w320) -> ()
        n235 = global write "Meas_global.vi" "Analysis type array"(w327) -> ()
        n236 = global write "Meas_global.vi" "Analysis Info cluster"(w325) -> ()
        n237 = global write "Meas_global.vi" "Velocity Cluster Array"(w319) -> ()
        n238 = property on="Plot 1" class="Ring (strict)"("Strings []"=w324) -> ()  [unwired: 2 in, 2 out]
        n239 = property on="Plot 1" class="Ring (strict)"("Strings []"=w324) -> ()  [unwired: 2 in, 2 out]
        n240 = property on="Plot 2" class="Ring (strict)"("Strings []"=w324) -> ()  [unwired: 2 in, 2 out]
        n241 = property on="Plot 2" class="Ring (strict)"("Strings []"=w324) -> ()  [unwired: 2 in, 2 out]
      }
      frame #11 {
        n242 = global read "Meas_global.vi" "Analysis Info cluster"() -> (w351:T20[])
        n243 = for {
          tunnel: w351 -> [w355] mode=indexing
          tunnel: [w354] -> w350 mode=indexing
          tunnel: [w353] -> w341
          i -> [w353]
          n244 = Unbundle By Name(w355) -> ("Inst name"=w354:string)
        }
        n245 = Greater Than 0?(x=w341) -> (x > 0?=w340:bool)
        n246 = Select(t="Correlate?", s=w340, f=T6."Cross correlation off" ("Correlate?")) -> (s? t:f=w342:T6)
        n247 = case shown="\"Correlate without activating panel\"" w342 {
          tunnel: w350 -> [_ w360 w362]
          tunnel: [w357 w359 w361] -> w339
          frame "Cross correlation off" {
            n248 = Initialize Array(0) -> (w357:i32[][])  [unwired: 2 out]
          }
          frame "Show correlation panel" {
            w358 = FALSE  # OK
            n249 = call "Correlation_Display.vi"("Inst names"=w360, "OK"=w358) -> ("correlation array"=w359:i32[][])  [unwired: 2 in, 2 out]
          }
          frame "Correlate without activating panel" {
            n250 = call "Correlation_Display.vi"("Inst names"=w362, "OK"=TRUE) -> ("correlation array"=w361:i32[][])  [unwired: 2 in, 2 out]
          }
        }
        n251 = global read "Meas_global.vi" "Position"() -> (w349:T7)
        n252 = local write "Position"(w349) -> ()
        n253 = global write "Meas_global.vi" "correlate"(w339) -> ()
        n254 = Array Size(array=w339) -> (size(s)=w348:i32[])
        n255 = Index Array(array=w348, index=0) -> (element=w346:i32)
        n256 = Equal To 0?(x=w346) -> (x = 0?=w345:bool)
        n257 = case shown="True" w345 {
          frame False {
          }
          frame True {
            n258 = local write "Correlate?"(T6."Cross correlation off" ("Correlate?")) -> ()
          }
        }
      }
      frame #12 {
        n259 = stacked-sequence {
          seq-local: [w370 _] -> [_ w392]
          tunnel: w364 -> [w369 _]
          frame #0 {
            n260 = call "LDA+_An_Analysis_mode.vi"("Second Graph"="Second Graph", "First Graph"="First Graph") -> ("Second Graph out"=w365:T3, "First Graph out"=w367:T3)  [unwired: 6 out]
            n261 = case shown="False" w369 {
              tunnel: [w380 w391] -> w368
              tunnel: w367 -> [w379 w391]
              tunnel: [w378 w390] -> w366
              tunnel: w365 -> [w377 w390]
              frame False {
                w375 = Graph_Type."Show no graph" ("Plot Type")
                n262 = Unbundle By Name(w379) -> ("Save graph"=w381:u16)
                n263 = Unbundle By Name(w377) -> ("Save graph"=w376:u16)
                n264 = case shown="0, Default" w381 {
                  tunnel: [w387 w389] -> w380
                  tunnel: w379 -> [w388 w389]
                  tunnel: w375 -> [w386 _]
                  frame 0, Default {
                    n265 = Bundle By Name(cluster=w388, "Plot Type"=w386) -> (w387:T3)
                  }
                  frame 1 {
                  }
                }
                n266 = case shown="0, Default" w376 {
                  tunnel: [w383 w385] -> w378
                  tunnel: w377 -> [w384 w385]
                  tunnel: w375 -> [w382 _]
                  frame 0, Default {
                    n267 = Bundle By Name(cluster=w384, "Plot Type"=w382) -> (w383:T3)
                  }
                  frame 1 {
                  }
                }
              }
              frame True {
              }
            }
            n268 = local write "Second Graph"(w366) -> ()
            n269 = local write "First Graph"(w368) -> ()
            n270 = global write "Meas_global.vi" "Second Graph"(w366) -> ()
            n271 = global write "Meas_global.vi" "First Graph"(w368) -> ()
            n272 = Unbundle By Name(w366) -> ("Plot Type"=w374:T2)
            n273 = Unbundle By Name(w368) -> ("Plot Type"=w373:T2)
            n274 = Build Array(w373, w374) -> (w370:T2[])
          }
          frame #1 {
            n275 = global read "Meas_global.vi" "Insts for plotting"() -> (w393:u16[][])
            n276 = for {
              tunnel: w393 -> [w395] mode=indexing
              tunnel: w392 -> [w394] mode=indexing
              i -> [w396]
              n277 = stacked-sequence {
                seq-local: [w399 _] -> [_ w409]
                seq-local: [w400 _] -> [_ w408]
                tunnel: w396 -> [_ w412]
                tunnel: w395 -> [w398 _]
                tunnel: w394 -> [_ w404]
                frame #0 {
                  n278 = property on="Plot 1" class="Ring (strict)"() -> ("Strings []"=w397:string[])  [unwired: 2 in, 2 out]
                  n279 = Array To Cluster(array=w398) -> (cluster=w403:T30)
                  n280 = Unbundle(w403) -> ("Insts for plotting[0]"=w402:u16, "Insts for plotting[1]"=w401:u16)
                  n281 = Index Array(array=w397, index=w402) -> (element=w399:string)
                  n282 = Index Array(array=w397, index=w401) -> (element=w400:string)
                }
                frame #1 {
                  n283 = case shown="\"Auto-Corr\"" w404 {
                    tunnel: [u8 0 u8 0 u8 0 u8 0 u8 0 u8 1 u8 0] -> w416
                    tunnel: [u8 0 u8 0 u8 0 u8 0 u8 1 u8 1 u8 0] -> w415
                    tunnel: [u8 0 u8 0 u8 0 u8 0 u8 1 u8 1 u8 0] -> w414
                    tunnel: [u8 0 u8 0 u8 0 u8 0 u8 1 u8 0 u8 0] -> w413
                    tunnel: [FALSE TRUE TRUE TRUE TRUE TRUE TRUE] -> w407
                    tunnel: [u8 0 u8 0 u8 0 u8 2 u8 0 u8 0 u8 2] -> w406
                    tunnel: [u8 0 u8 4 u8 1 u8 2 u8 0 u8 0 u8 1] -> w405
                    frame "Show no graph" {
                    }
                    frame "Voltage trace" {
                    }
                    frame "Velocity trace" {
                    }
                    frame "Vel histogram" {
                    }
                    frame "Spectrum" {
                    }
                    frame "f.E(f) v Log f" {
                    }
                    frame "Auto-Corr" {
                    }
                  }
                  n284 = case shown="0, Default" w412 {
                    tunnel: w407 -> [w427 w438]
                    tunnel: w416 -> [w426 w437]
                    tunnel: w415 -> [w425 w436]
                    tunnel: w414 -> [w424 w435]
                    tunnel: w413 -> [w423 w434]
                    tunnel: u32 0 -> [w422 w433]
                    tunnel: u32 1 -> [w421 w431]
                    tunnel: w409 -> [w420 w432]
                    tunnel: w408 -> [w419 w430]
                    tunnel: w406 -> [w418 w429]
                    tunnel: w405 -> [w417 w428]
                    frame 0, Default {
                      n285 = property on="First plot" class="WFGraph (strict)"("Visible"=w427, "X Scale.Format & Precision:Format"=w426, "X Scale.Mapping Mode"=w425, "Y Scale.Format & Precision:Format"=w424, "Y Scale.Mapping Mode"=w423, "Active Plot"=w422, "Plot.Plot Name"=w420, "Active Plot"=w421, "Plot.Plot Name"=w419, "X Scale.Format & Precision:Precision"=w418, "Y Scale.Format & Precision:Precision"=w417) -> ()  [unwired: 2 in, 2 out]
                    }
                    frame 1 {
                      n286 = property on="2nd plot" class="WFGraph (strict)"("Visible"=w438, "X Scale.Format & Precision:Format"=w437, "X Scale.Mapping Mode"=w436, "Y Scale.Format & Precision:Format"=w435, "Y Scale.Mapping Mode"=w434, "Active Plot"=w433, "Plot.Plot Name"=w432, "Active Plot"=w431, "Plot.Plot Name"=w430, "X Scale.Format & Precision:Precision"=w429, "Y Scale.Format & Precision:Precision"=w428) -> ()  [unwired: 2 in, 2 out]
                    }
                  }
                }
              }
            }
          }
        }
      }
      frame #13 {
        n287 = local read "Second Graph"() -> (w499:T3)
        n288 = local read "First Graph"() -> (w498:T3)
        n289 = Unbundle By Name(w498) -> ("Plot 1"=w491:u16, "Plot 2"=w492:u16)
        n290 = Unbundle By Name(w499) -> ("Plot 1"=w493:u16, "Plot 2"=w494:u16)
        n291 = Build Array(w491, w492) -> (w495:u16[])
        n292 = Build Array(w493, w494) -> (w496:u16[])
        n293 = global read "Meas_global.vi" "Analysis Info cluster"() -> (w500:T20[])
        n294 = Decrement(x=w495) -> (x-1=w489:u16[])
        n295 = Decrement(x=w496) -> (x-1=w497:u16[])
        n296 = for {
          tunnel: w500 -> [w508]
          tunnel: w489 -> [w507] mode=indexing
          shift-right: [w501] -> _
          shift-left: u32 0 -> [w503]
          i -> [w502]
          n297 = Index Array(array=w508, index=w507) -> (element=w509:T20)
          n298 = Unbundle By Name(w509) -> ("Colour"=w504:u32)
          n299 = Equal?(x=w504, y=w503) -> (x = y?=w506:bool)
          n300 = Select(t=u32 13434624, s=w506, f=w504) -> (s? t:f=w501:u32)
          n301 = property on="First plot" class="WFGraph (strict)"("Active Plot"=w502, "Plot.Plot Color"=w501, "Plot.Fill/Point Color"=w501) -> ()  [unwired: 2 in, 2 out]
        }
        n302 = for {
          tunnel: w500 -> [w517]
          tunnel: w497 -> [w516] mode=indexing
          shift-right: [w512] -> _
          shift-left: u32 0 -> [w510]
          i -> [w515]
          n303 = Index Array(array=w517, index=w516) -> (element=w518:T20)
          n304 = Unbundle By Name(w518) -> ("Colour"=w511:u32)
          n305 = Equal?(x=w511, y=w510) -> (x = y?=w514:bool)
          n306 = Select(t=u32 13434624, s=w514, f=w511) -> (s? t:f=w512:u32)
          n307 = property on="2nd plot" class="WFGraph (strict)"("Active Plot"=w515, "Plot.Plot Color"=w512, "Plot.Fill/Point Color"=w512) -> ()  [unwired: 2 in, 2 out]
        }
      }
      frame #14 {
        n308 = global read "DataTranslation_global.vi" "Different Sampling Freq per block"() -> (w519:bool)
        n309 = global read "Meas_global.vi" "Remote control"() -> (w528:bool)
        n310 = global read "Meas_global.vi" "Post Process"() -> (w531:T5)
        n311 = global read "Meas_global.vi" "PWA Data"() -> (w520:T31)
        n312 = case shown="\"One Ch PWA\"" w520 {
          tunnel: [w532 w537] -> w522
          frame "No PWA Data" {
            n313 = local read "Desired Sampling freq (Hz)"() -> (w534:dbl)
            n314 = local read "No of samples"() -> (w533:i32)
            n315 = Divide(x=w533, y=w534) -> (x/y=w532:dbl)
          }
          frame "One Ch PWA" {
            n316 = local read "No of samples"() -> (w535:i32)
            n317 = global read "PWAtasksGLOBAL.vi" "PWA Freq. (Hz)"() -> (w536:dbl)
            n318 = global write "PWAtasksGLOBAL.vi" "PWA No. of Samples"(w535) -> ()
            n319 = Divide(x=w535, y=w536) -> (x/y=w537:dbl)
          }
        }
        n320 = global read "Meas_global.vi" "Averaging time (min)"() -> (w526:dbl)
        n321 = Equal?(x=Setup."Run Program" ("setup"), y=w525) -> (x = y?=w523:bool)
        n322 = Equal?(x=Post_Process."Take New Data" ("Post Process"), y=w531) -> (x = y?=w527:bool)
        n323 = Compound Arithmetic op=AND(invert w519, w527, invert w521, invert w528, w523) -> (w529:bool)
        n324 = case shown="True" w529 {
          tunnel: w526 -> [_ w544]
          tunnel: w522 -> [_ w543]
          tunnel: w520 -> [_ w538]
          frame False {
          }
          frame True {
            n325 = global read "Meas_global.vi" "Board type"() -> (w541:T13)
            n326 = Equal?(x=w541, y=Board_Types."Simulate" ("Board type")) -> (x = y?=w540:bool)
            n327 = case shown="False" w540 {
              tunnel: w544 -> [w554 _]
              tunnel: w543 -> [w547 _]
              tunnel: [w546 1 ("No of Blocks")] -> w539
              tunnel: w538 -> [w545 _]
              frame False {
                n328 = Multiply(x=w554, y=60.0) -> (x*y=w552:dbl)
                n329 = global read "Meas_global.vi" "LDA data"() -> (w556:enum16{"No LDA data", "Take LDA data"})
                n330 = Equal?(x=enum16{"No LDA data", "Take LDA data"}."Take LDA data" ("LDA data"), y=w556) -> (x = y?=w550:bool)
                n331 = Divide(x=w552, y=w547) -> (x/y=w551:dbl)
                n332 = Round Toward +Infinity(x=w551) -> (ceil(x): smallest int >= x=w549:dbl)
                n333 = To Long Integer(number=w549) -> (32bit integer=w548:i32)
                n334 = case shown="\"No PWA Data\"" w545 {
                  tunnel: w550 -> [w560 _]
                  tunnel: w548 -> [w558 w561]
                  tunnel: [w557 w561] -> w546
                  frame "No PWA Data" {
                    n335 = Select(t=99999 ("No of Blocks"), s=w560, f=w558) -> (s? t:f=w557:i32)
                  }
                  frame "One Ch PWA" {
                  }
                }
              }
              frame True {
              }
            }
            n336 = global write "Meas_global.vi" "Requested No of blocks"(w539) -> ()
            n337 = local write "No of Blocks"(w539) -> ()
          }
        }
      }
      frame #15 {
        n338 = case shown="\"Run Program\"" w563 {
          frame "Run Program" {
            n339 = call "Read_calibration_files.vi"() -> ()  [unwired: 1 out]
            n340 = global write "Meas_global.vi" "Repeat Measurement?"(FALSE ("Repeat Measurement?")) -> ()
          }
          frame "Show Setup", Default {
          }
        }
      }
      frame #16 {
        n341 = global read "Meas_global.vi" "Raw data option"() -> (w568:enum16{"Save raw data", "Raw data not saved"})
        n342 = Get Date/Time In Seconds() -> (seconds since 1Jan1904=w569:timestamp)
        n343 = To Double Precision Float(number=w569) -> (double precision float=w566:dbl)
        n344 = global read "Meas_global.vi" "Post Process"() -> (w567:T5)
        n345 = case shown="\"Save Current Setup\"" w570 {
          tunnel: w568 -> [w573 _ _ _]
          tunnel: w567 -> [w572 _ w605 w614]
          frame "Run Program" {
            n346 = case shown="\"Take New Data\"" w572 {
              tunnel: w573 -> [w574 _]
              frame "Take New Data" {
                n347 = case shown="\"Raw data not saved\"" w574 {
                  frame "Save raw data" {
                  }
                  frame "Raw data not saved" {
                    w582 = FALSE  # Lock File
                    w579 = FALSE  # advisory dialog? (display:T)
                    w578 = FALSE  # append to file? (new file:F)
                    n348 = global read "Meas_global.vi" "Remote control"() -> (w580:bool)
                    n349 = call "Create_setup_string.vi"() -> ("Setup String"=w583:string)  [unwired: 1 out]
                    n350 = case shown="False" w580 {
                      tunnel: ["Current_Setup.xls" ("Setup filename") w585] -> w575
                      frame False {
                      }
                      frame True {
                        n351 = local read "Setup filename"() -> (w585:string)
                      }
                    }
                    n352 = call "Add_length_to_string.vi"("String in"=w583) -> ("String out"=w581:string)
                    n353 = call "Setup_Filepath.vi"("Setup File Type"=Setup_Filetype."Measurement Setups", "Filename in"=w575) -> ("Filename Out"=w576:path)  [unwired: 1 out]
                    n354 = call "Write_Characters_To_File.vi"("file path (dialog if empty)"=w576, "advisory dialog? (display:T)"=w579, "character string"=w581, "append to file? (new file:F)"=w578, "Lock File"=w582) -> ()  [unwired: 4 out]
                  }
                }
              }
              frame "Post Process Raw Data File" {
              }
            }
          }
          frame "Save Current Setup" {
            n355 = stacked-sequence {
              seq-local: [w588 _] -> [_ w591]
              seq-local: [w587 _] -> [_ w590]
              frame #0 {
                w589 = FALSE  # Save New File?
                n356 = call "Save_current_setup.vi"("Save New File?"=w589, "Setup File Type"=Setup_Filetype."Measurement Setups") -> ("Cancelled?"=w587:bool, "Saved filepath"=w588:path)  [unwired: 2 out]
              }
              frame #1 {
                n357 = case shown="False" w590 {
                  tunnel: w591 -> [w597 _]
                  frame False {
                    w594 = "Initial Probe positions" ("File Label")
                    w602 = FALSE  # append to file? (new file:F)
                    w603 = FALSE  # advisory dialog? (display:T)
                    w604 = FALSE  # Lock File
                    n358 = call "Input_Instrument_Positions.vi"("Filepath to Save"=w597) -> ("Output string"=w596:string)  [unwired: 1 out]
                    n359 = call "Create_setup_string.vi"() -> ("Setup String"=w595:string)  [unwired: 1 out]
                    n360 = call "Get_string_subset.vi"("String to split"=w596, "File Label"=w594) -> ("Output string"=w593:string)  [unwired: 2 in, 1 out]
                    n361 = call "Replace_data_in_Label_str.vi"("New data string"=w593, "Input string"=w595, "Variable name"=w594) -> ("Appended string"=w592:string)
                    n362 = call "Replace_data_in_setup_string.vi"("New data string"="", "Input string"=w592, "Variable name"="Comments") -> ("Appended string"=w598:string)
                    n363 = call "Add_length_to_string.vi"("String in"=w598) -> ("String out"=w601:string)
                    n364 = call "Write_Characters_To_File.vi"("file path (dialog if empty)"=w597, "advisory dialog? (display:T)"=w603, "character string"=w601, "append to file? (new file:F)"=w602, "Lock File"=w604) -> ()  [unwired: 4 out]
                  }
                  frame True {
                  }
                }
              }
            }
          }
          frame "Show Setup" {
            n365 = case shown="\"Take New Data\"" w605 {
              frame "Take New Data" {
                w610 = FALSE  # append to file? (new file:F)
                w611 = FALSE  # advisory dialog? (display:T)
                w612 = FALSE  # Lock File
                n366 = call "Create_setup_string.vi"() -> ("Setup String"=w613:string)  [unwired: 1 out]
                n367 = call "Add_length_to_string.vi"("String in"=w613) -> ("String out"=w609:string)
                n368 = call "Setup_Filepath.vi"("Setup File Type"=Setup_Filetype."Measurement Setups", "Filename in"="Current_Setup.xls" ("Setup filename")) -> ("Filename Out"=w607:path)  [unwired: 1 out]
                n369 = call "Write_Characters_To_File.vi"("file path (dialog if empty)"=w607, "advisory dialog? (display:T)"=w611, "character string"=w609, "append to file? (new file:F)"=w610, "Lock File"=w612) -> ()  [unwired: 4 out]
              }
              frame "Post Process Raw Data File" {
              }
            }
          }
          frame "Setup Front Panel" {
            n370 = case shown="\"Take New Data\"" w614 {
              frame "Take New Data" {
                w619 = FALSE  # append to file? (new file:F)
                w620 = FALSE  # advisory dialog? (display:T)
                w621 = FALSE  # Lock File
                n371 = call "Create_setup_string.vi"() -> ("Setup String"=w622:string)  [unwired: 1 out]
                n372 = call "Add_length_to_string.vi"("String in"=w622) -> ("String out"=w618:string)
                n373 = call "Setup_Filepath.vi"("Setup File Type"=Setup_Filetype."Measurement Setups", "Filename in"="Current_Setup.xls" ("Setup filename")) -> ("Filename Out"=w616:path)  [unwired: 1 out]
                n374 = call "Write_Characters_To_File.vi"("file path (dialog if empty)"=w616, "advisory dialog? (display:T)"=w620, "character string"=w618, "append to file? (new file:F)"=w619, "Lock File"=w621) -> ()  [unwired: 4 out]
              }
              frame "Post Process Raw Data File" {
              }
            }
          }
        }
        n375 = call "Program_Active.vi"() -> ()  [unwired: 1 in]
        n376 = global write "Meas_global.vi" "Actual Measurement time (min)"(0.0 ("Max Measurement time (min)")) -> ()
        n377 = global write "Meas_global.vi" "Current Block No"(0 ("Current Block No")) -> ()
      }
      frame #17 {
        n378 = case shown="\"Run Program\"" w626 {
          tunnel: w623 -> [w628 _]
          tunnel: w625 -> [_ w815]
          tunnel: w624 -> [w627 _]
          frame "Run Program" {
            # "PWA"
            # "LDA"
            # "An"
            n379 = stacked-sequence {
              seq-local: [w636 _] -> [_ w658]
              seq-local: [w635 _] -> [_ w657]
              seq-local: [w634 _] -> [_ w656]
              seq-local: [w632 _] -> [_ w655]
              seq-local: [w630 _] -> [_ w652]
              seq-local: [w629 _] -> [_ w651]
              tunnel: w628 -> [_ w654]
              tunnel: w627 -> [_ w653]
              frame #0 {
                n380 = global read "Trav_pos_global.vi" "Dummy Measurement?"() -> (w631:bool)
                n381 = case shown="False" w631 {
                  tunnel: [w643 u16[][] [] ("LDA Binary output")] -> w636
                  tunnel: [w642 w645] -> w635
                  tunnel: [w641 dbl[][] [] ("Voltage output")] -> w634
                  tunnel: [w640 TRUE ("EOF?")] -> w633
                  tunnel: [w639 T15 {"Started"=0.0, "Ended"=0.0, "Analogue Frequency Hz"=1000.0} ("Block Timings")] -> w632
                  tunnel: [w638 w645] -> w630
                  tunnel: [w637 ""] -> w629
                  frame False {
                    n382 = call "Get_data.vi"() -> ("EOF? and Error status"=w640:bool, "Voltage output"=w641:dbl[][], "Analogue Binary"=w642:i16[][], "LDA Binary output"=w643:u16[][], "Block Timings"=w639:T15, "PWA Binary"=w638:i16[][], "Block Header"=w637:string)  [unwired: 5 out]
                  }
                  frame True {
                    w645 = i16[][] [] ("Analogue Binary")
                  }
                }
                n383 = case shown="True" w633 {
                  frame False {
                  }
                  frame True {
                    n384 = local write "No of Blocks"(1 ("No of Blocks")) -> ()
                  }
                }
              }
              frame #1 {
                n385 = while {
                  tunnel: w654 -> [w664]
                  shift-left: w655 -> [w665]
                  shift-right: [w666] -> _
                  shift-left: w656 -> [w670]
                  shift-right: [w673] -> _
                  shift-left: w657 -> [w671]
                  shift-right: [w674] -> _
                  shift-left: w658 -> [w672]
                  shift-right: [w675] -> _
                  tunnel: w653 -> [w663]
                  shift-right: [w662] -> _
                  shift-left: w652 -> [w661]
                  shift-right: [w660] -> _
                  shift-left: w651 -> [w659]
                  i -> [w667]
                  stop <- w676 continue-if-true
                  n386 = Increment(x=w667) -> (x+1=w677:i32)
                  n387 = stacked-sequence {
                    seq-local: [_ _ _ _ _ "Block average display control" _ _ _ _] -> [_ _ _ _ _ _ w772 _ _ _]
                    seq-local: [_ _ _ _ _ _ w769 _ _ _] -> [_ _ _ _ _ _ _ w783 _ _]
                    seq-local: [w713 _ _ _ _ _ _ _ _ _] -> [_ w719 _ _ w755 _ _ _ _ w813]
                    seq-local: [_ _ w724 _ _ _ _ _ _ _] -> [_ _ _ _ w753 _ _ _ _ _]
                    seq-local: [_ _ _ w745 _ _ _ _ _ _] -> [_ _ _ _ w754 _ _ _ _ _]
                    tunnel: w677 -> [w712 _ _ _ w757 w765 _ _ _ _]
                    tunnel: [_ _ _ _ _ _ _ _ _ w813] -> w676
                    tunnel: w667 -> [_ _ _ _ _ _ _ _ _ _]
                    tunnel: w672 -> [_ _ _ w743 _ _ _ _ _ _]
                    tunnel: w671 -> [_ _ _ w742 _ _ _ _ _ _]
                    tunnel: w670 -> [_ _ _ w749 _ _ _ _ _ _]
                    tunnel: "stop" -> [w715 _ _ _ _ _ _ _ _ _]
                    tunnel: "No of Blocks" -> [w714 _ _ _ _ _ _ _ _ _]
                    tunnel: w665 -> [_ _ _ w747 _ _ _ _ _ _]
                    tunnel: w664 -> [_ _ w723 w744 _ _ _ _ _ _]
                    tunnel: w663 -> [_ _ w725 _ _ _ _ _ _ _]
                    tunnel: w661 -> [_ _ _ w741 _ _ _ _ _ _]
                    tunnel: w659 -> [w711 _ _ _ _ _ _ _ _ _]
                    frame #0 {
                      n388 = global write "Plug_in_data_global.vi" "Block Header"(w711) -> ()
                      n389 = Less Or Equal?(x=w714, y=w712) -> (x <= y?=w717:bool)
                      n390 = Or(x=w715, y=w717) -> (x .or. y?=w716:bool)
                      n391 = global write "Meas_global.vi" "Current Block No"(w712) -> ()
                      n392 = Not(x=w716) -> (.not. x?=w713:bool)
                    }
                    frame #1 {
                      n393 = call "Program_Active.vi"() -> ()  [unwired: 1 in]
                      n394 = call "Text_without_format.vi"("Input string"="Comments") -> ("Output string"=w720:string)
                      n395 = global write "Meas_global.vi" "Position"("Position") -> ()
                      n396 = local write "Comments"(w720) -> ()
                      n397 = global write "Meas_global.vi" "Comments"(w720) -> ()
                      n398 = Not(x=w719) -> (.not. x?=w718:bool)
                      n399 = global write "Meas_global.vi" "Processing last block?"(w718) -> ()
                      n400 = global write "PWAtasksGLOBAL.vi" "STOP"(w718) -> ()
                    }
                    frame #2 {
                      n401 = case shown="False" w723 {
                        tunnel: w725 -> [w737 _]
                        tunnel: [w726 FALSE] -> w724
                        frame False {
                          w734 = 1.5  # To allow for overhead
                          n402 = Get Date/Time In Seconds() -> (seconds since 1Jan1904=w739:timestamp)
                          n403 = global read "Meas_global.vi" "Averaging time (min)"() -> (w733:dbl)
                          n404 = To Double Precision Float(number=w739) -> (double precision float=w738:dbl)
                          n405 = Subtract(x=w738, y=w737) -> (x-y=w736:dbl)
                          n406 = global read "Meas_global.vi" "LDA data"() -> (w730:enum16{"No LDA data", "Take LDA data"})
                          n407 = Divide(x=w736, y=60.0 ("To convert to minutes")) -> (x/y=w732:dbl)
                          n408 = Equal?(x=enum16{"No LDA data", "Take LDA data"}."Take LDA data" ("LDA data"), y=w730) -> (x = y?=w727:bool)
                          n409 = Multiply(x=w734, y=w733) -> (x*y=w731:dbl)
                          n410 = Greater?(x=w732, y=w731) -> (0:w728:bool)
                          n411 = And(x=w727, y=w728) -> (x .and. y?=w726:bool)
                        }
                        frame True {
                        }
                      }
                    }
                    frame #3 {
                      n412 = call "Process_data.vi"("PWA Binary"=w741, "Analogue Binary"=w742, "LDA Binary output"=w743, "Analogue volts"=w749, "Measurement top level?"=w744, "Block Timings"=w747) -> ("Vel stat display"=→"Statistics":string[][], "First Plot data"=→"First plot":cluster{"Xo":dbl, "Delta X":dbl, dbl[]}[], "Second Plot data"=→"2nd plot":cluster{"Xo":dbl, "Delta X":dbl, dbl[]}[], "Max Measurement time up"=w745:bool)
                    }
                    frame #4 {
                      n413 = global read "Meas_global.vi" "stop"() -> (w752:bool)
                      n414 = Compound Arithmetic op=OR(w752, w753, w754) -> (w751:bool)
                      n415 = And(x=w755, y=w751) -> (x .and. y?=w756:bool)
                      n416 = case shown="True" w756 {
                        tunnel: w757 -> [_ w758]
                        frame False {
                        }
                        frame True {
                          n417 = Increment(x=w758) -> (x+1=w759:i32)
                          n418 = local write "No of Blocks"(w759) -> ()
                        }
                      }
                    }
                    frame #5 {
                      n419 = global read "Meas_global.vi" "Actual Measurement time (min)"() -> (→"Measurement time (min)":dbl)
                      n420 = global read "Meas_global.vi" "Actual Sampling rate (Hz)"() -> (→"Actual Sampling freq":dbl)
                      n421 = call "Display_blocks.vi"("Block No"=w765, "Block average display"="Block average display control") -> ("u^4"=→"u^4":dbl[][], "u^3"=→"u^3":dbl[][], "uv"=→"uv":dbl[][], "u^2"=→"u^2" →"Array u^2":dbl[][], "U"=→"U" →"Array U":dbl[][])  [unwired: 4 out]
                    }
                    frame #6 {
                      n422 = global read "Meas_global.vi" "Analysis Info cluster"() -> (w771:T20[])
                      n423 = for {
                        tunnel: w772 -> [w777] mode=indexing
                        shift-right: [w773] -> w769
                        shift-left: u32[] [] -> [w774]
                        tunnel: w771 -> [w776] mode=indexing
                        n424 = Unbundle By Name(w777) -> ("Include"=w775:bool)
                        n425 = case shown="True" w775 {
                          tunnel: w776 -> [_ w782]
                          tunnel: w774 -> [w778 w780]
                          tunnel: [w778 w779] -> w773
                          frame False {
                          }
                          frame True {
                            n426 = Unbundle By Name(w782) -> ("Colour"=w781:u32)
                            n427 = Build Array (concatenate)(w780, w781) -> (w779:u32[])
                          }
                        }
                      }
                    }
                    frame #7 {
                      n428 = for {
                        tunnel: w783 -> [w784] mode=indexing
                        i -> [w785]
                        n429 = property on="U" class="WFGraph (strict)"("Active Plot"=w785, "Plot.Plot Color"=w784, "Plot.Fill/Point Color"=w784) -> ()  [unwired: 2 in, 2 out]
                        n430 = property on="u^3" class="WFGraph (strict)"("Active Plot"=w785, "Plot.Plot Color"=w784, "Plot.Fill/Point Color"=w784) -> ()  [unwired: 2 in, 2 out]
                        n431 = property on="u^4" class="WFGraph (strict)"("Active Plot"=w785, "Plot.Plot Color"=w784, "Plot.Fill/Point Color"=w784) -> ()  [unwired: 2 in, 2 out]
                        n432 = property on="u^2" class="WFGraph (strict)"("Active Plot"=w785, "Plot.Plot Color"=w784, "Plot.Fill/Point Color"=w784) -> ()  [unwired: 2 in, 2 out]
                      }
                    }
                    frame #8 {
                      n433 = case shown="True" "Pause" {
                        frame False {
                        }
                        frame True {
                          n434 = global read "Meas_global.vi" "Post Process"() -> (w787:T5)
                          n435 = case shown="\"Take New Data\"" w787 {
                            frame "Take New Data" {
                              n436 = call "Program_Active_Client.vi"("Mode"=enum16{"Program Active", "Traverse Level State"}."Program Active", "Time till next contact (Sec)"=12000.0, "Traverse level State"=Traverse_Level_State."Running") -> ()  [unwired: 3 out]
                              n437 = while {
                                i -> [w794]
                                stop <- w795 continue-if-true
                                n438 = Quotient & Remainder(x=w794, y=10) -> (x-y*floor(x/y)=w792:i32)  [unwired: 1 out]
                                n439 = Equal To 0?(x=w792) -> (x = 0?=w791:bool)
                                n440 = stacked-sequence {
                                seq-local: [_ w797 _ _] -> [_ _ w799 _]
                                tunnel: [_ w797 _ _] -> w795
                                tunnel: w791 -> [_ _ _ w801]
                                frame #0 {
                                "Pause message" <- "Measurement Program Paused!!!!" ("Pause message")
                                }
                                frame #1 {
                                n441 = global write "Trav_pos_global.vi" "Paused During Row?"(TRUE ("Paused During Row?")) -> ()
                                n442 = local read "Pause"() -> (w797:bool)
                                }
                                frame #2 {
                                n443 = property on="Pause message" class="Str"("Blinking"=w799, "Visible"=w799) -> ()  [unwired: 2 in, 2 out]
                                n444 = Wait Until Next ms Multiple(millisecond multiple=u32 1000) -> ()  [unwired: 1 out]
                                }
                                frame #3 {
                                n445 = case shown="False" w801 {
                                frame False {
                                }
                                frame True {
                                n446 = Current VI's Path() -> (path=w802:path)
                                n447 = call "Bring_to_front.vi"("path"=w802) -> ()
                                }
                                }
                                }
                                }
                              }
                            }
                            frame "Post Process Raw Data File" {
                              n448 = stacked-sequence {
                                seq-local: [_ w805 _ _] -> [_ _ _ w812]
                                frame #0 {
                                n449 = property on="PP next block" class="Bool (strict)"("Visible"=TRUE) -> ()  [unwired: 2 in, 2 out]
                                n450 = local write "PP next block"(FALSE ("PP next block")) -> ()
                                }
                                frame #1 {
                                n451 = while {
                                tunnel: [w809] -> w805
                                stop <- w806 stop-if-true
                                n452 = local read "stop"() -> (w809:bool)
                                n453 = local read "Pause"() -> (w807:bool)
                                n454 = Compound Arithmetic op=OR(w809, "PP next block", invert w807) -> (w806:bool)
                                n455 = case shown="False" w806 {
                                frame False {
                                n456 = Wait (ms)(milliseconds to wait=u32 200) -> ()  [unwired: 1 out]
                                }
                                frame True {
                                }
                                }
                                }
                                }
                                frame #2 {
                                n457 = property on="PP next block" class="Bool (strict)"("Visible"=FALSE) -> ()  [unwired: 2 in, 2 out]
                                }
                                frame #3 {
                                n458 = Stop(stop? (T)=w812) -> ()
                                }
                              }
                            }
                          }
                        }
                      }
                    }
                    frame #9 {
                      n459 = global read "Meas_global.vi" "Diagnostic info"() -> (→"BSA Diagnostic info":string[][])
                    }
                  }
                  n460 = stacked-sequence {
                    seq-local: [w679 _ _] -> [_ w689 _]
                    seq-local: [_ w688 _] -> [_ _ w709]
                    tunnel: [_ w692 _] -> w675
                    tunnel: [_ w691 _] -> w674
                    tunnel: [_ w690 _] -> w673
                    tunnel: "No of Blocks" -> [w684 _ _]
                    tunnel: "stop" -> [w682 _ _]
                    tunnel: w667 -> [w680 _ w708]
                    tunnel: [_ w687 _] -> w666
                    tunnel: [_ w686 _] -> w662
                    tunnel: [_ w685 _] -> w660
                    frame #0 {
                      n461 = Increment(x=w680) -> (x+1=w678:i32)
                      "Current Block No" <- w678
                      n462 = Less Or Equal?(x=w684, y=w678) -> (x <= y?=w683:bool)
                      n463 = Or(x=w683, y=w682) -> (x .or. y?=w681:bool)
                      n464 = Not(x=w681) -> (.not. x?=w679:bool)
                      n465 = global write "Meas_global.vi" "Current Block No"(w678) -> ()
                    }
                    frame #1 {
                      n466 = case shown="True" w689 {
                        tunnel: [u16[][] [] ("LDA Binary output") w705] -> w692
                        tunnel: [w694 w704] -> w691
                        tunnel: [dbl[][] [] ("Voltage output") w703] -> w690
                        tunnel: [FALSE ("EOF?") w702] -> w688
                        tunnel: [T15 {"Started"=0.0, "Ended"=0.0, "Analogue Frequency Hz"=200.0} ("Block Timings") w701] -> w687
                        tunnel: [w694 w700] -> w686
                        tunnel: ["" w699] -> w685
                        frame False {
                          w694 = i16[][] [] ("Analogue Binary")
                        }
                        frame True {
                          n467 = call "Get_data.vi"() -> ("EOF? and Error status"=w702:bool, "Voltage output"=w703:dbl[][], "Analogue Binary"=w704:i16[][], "LDA Binary output"=w705:u16[][], "Block Timings"=w701:T15, "PWA Binary"=w700:i16[][], "Block Header"=w699:string)  [unwired: 5 out]
                        }
                      }
                    }
                    frame #2 {
                      n468 = Increment(x=w708) -> (x+1=w706:i32)
                      n469 = Increment(x=w706) -> (x+1=w707:i32)
                      n470 = case shown="True" w709 {
                        tunnel: w707 -> [_ w710]
                        frame False {
                        }
                        frame True {
                          n471 = local write "No of Blocks"(w710) -> ()
                        }
                      }
                    }
                  }
                }
              }
            }
          }
          frame "Setup Front Panel", Default {
            n472 = stacked-sequence {
              seq-local: [w816 _ _ _ _ _ _] -> [_ _ _ _ _ w890 _]
              seq-local: [_ w822 _ _ _ _ _] -> [_ _ _ _ _ w889 _]
              seq-local: [_ _ _ w853 _ _ _] -> [_ _ _ _ _ w888 _]
              seq-local: [_ _ _ _ w866 _ _] -> [_ _ _ _ _ w886 _]
              seq-local: [_ w821 _ _ _ _ _] -> [_ _ _ _ _ _ w903]
              seq-local: [_ _ w847 _ _ _ _] -> [_ _ _ _ _ w885 _]
              tunnel: w815 -> [_ w823 _ _ _ _ _]
              frame #0 {
                n473 = Build Array("Name", "Channel", "High limit", "Low limit") -> (w816:string[])
              }
              frame #1 {
                n474 = global read "Meas_global.vi" "LDA data"() -> (w821:enum16{"No LDA data", "Take LDA data"})
                n475 = case shown="\"Take LDA data\"" w821 {
                  tunnel: w823 -> [_ w834]
                  tunnel: [string[][] [] w831] -> w822
                  frame "No LDA data" {
                  }
                  frame "Take LDA data" {
                    n476 = case shown="\"2D\"" w834 {
                      tunnel: [string[] [] w840] -> w832
                      frame "1D" {
                      }
                      frame "2D" {
                        n477 = global read "LDA_meas_global_2.vi" "Max Vel BSA2"() -> (w839:dbl)
                        n478 = global read "LDA_meas_global_2.vi" "Min Vel BSA2"() -> (w838:dbl)
                        n479 = global read "LDA_meas_global_2.vi" "Vel Comp BSA2"() -> (w841:string)
                        n480 = Format Into String(format string="%.1f m/s" ("Format String"), w838) -> (resulting string=w846:string)  [unwired: 2 in, 1 out]
                        n481 = Format Into String(format string="%.1f m/s" ("Format String"), w839) -> (resulting string=w845:string)  [unwired: 2 in, 1 out]
                        n482 = Build Array("LDA", w841, w845, w846) -> (w840:string[])
                      }
                    }
                    n483 = global read "LDA_meas_global_1.vi" "Max Vel BSA1"() -> (w826:dbl)
                    n484 = global read "LDA_meas_global_1.vi" "Vel Comp BSA1"() -> (w835:string)
                    n485 = global read "LDA_meas_global_1.vi" "Min Vel BSA1"() -> (w825:dbl)
                    n486 = Format Into String(format string="%.1f m/s" ("Format String"), w825) -> (resulting string=w827:string)  [unwired: 2 in, 1 out]
                    n487 = Format Into String(format string="%.1f m/s" ("Format String"), w826) -> (resulting string=w828:string)  [unwired: 2 in, 1 out]
                    n488 = Build Array("LDA", w835, w828, w827) -> (w833:string[])
                    n489 = Build Array(w833, w832) -> (w831:string[][])
                  }
                }
              }
              frame #2 {
                n490 = global read "Meas_global.vi" "PWA Data"() -> (w848:T31)
                n491 = case shown="\"One Ch PWA\"" w848 {
                  tunnel: [string[][] [] w850] -> w847
                  frame "No PWA Data" {
                  }
                  frame "One Ch PWA" {
                    n492 = Build Array("PWA") -> (w851:string[])
                    n493 = Build Array(w851) -> (w850:string[][])
                  }
                }
              }
              frame #3 {
                n494 = global read "Meas_global.vi" "Ch & spans"() -> (w854:T26[])
                n495 = for {
                  tunnel: w854 -> [w865] mode=indexing
                  tunnel: [w861] -> w853 mode=indexing
                  n496 = Unbundle By Name(w865) -> ("Var name"=w864:string, "Ch No"=w863:i16, "high limit (10V)"=w858:sgl, "low limit (-10V)"=w857:sgl)
                  n497 = Format Into String(format string="%.1f Volts" ("Format String"), w858) -> (resulting string=w856:string)  [unwired: 2 in, 1 out]
                  n498 = Format Into String(format string="%.1f Volts" ("Format String"), w857) -> (resulting string=w855:string)  [unwired: 2 in, 1 out]
                  n499 = Number To Decimal String(number=w863) -> (decimal integer string=w862:string)  [unwired: 1 out]
                  n500 = Build Array(w864, w862, w856, w855) -> (w861:string[])
                }
              }
              frame #4 {
                n501 = global read "Meas_global.vi" "Analysis Info cluster"() -> (w874:T20[])
                n502 = for {
                  tunnel: w874 -> [w884] mode=indexing
                  tunnel: [w883] -> w872 mode=indexing
                  n503 = Unbundle By Name(w884) -> ("Inst name"=w883:string)
                }
                n504 = global read "Meas_global.vi" "correlate"() -> (w873:i32[][])
                n505 = for {
                  tunnel: w873 -> [w879] mode=indexing
                  tunnel: w872 -> [w878]
                  tunnel: "Correlating" -> [w877]
                  tunnel: [w875] -> w867 mode=indexing
                  n506 = for {
                    tunnel: w879 -> [w882] mode=indexing
                    tunnel: w878 -> [w881]
                    tunnel: [w880] -> w876 mode=indexing
                    n507 = Index Array(array=w881, index=w882) -> (element=w880:string)
                  }
                  n508 = Build Array (concatenate)(w877, w876) -> (w875:string[])
                }
                n509 = Initialize Array("", 5 ("Dimension Size")) -> (w868:string[])
                n510 = Build Array (concatenate)(w868, w867) -> (w866:string[][])
              }
              frame #5 {
                n511 = Build Array (concatenate)(w890, w889, w885, w888, w886) -> (w887:string[][])
                n512 = local write "Statistics"(w887) -> ()
              }
              frame #6 {
                n513 = global read "Meas_global.vi" "Board type"() -> (w901:T13)
                n514 = global read "Meas_global.vi" "Continuous time trace?"() -> (w902:bool)
                n515 = Equal?(x=w901, y=Board_Types."ADC488" ("Board type")) -> (x = y?=w899:bool)
                n516 = case shown="\"Take LDA data\"" w903 {
                  tunnel: w899 -> [_ w907]
                  tunnel: [string[] [] w906] -> w895
                  frame "No LDA data" {
                  }
                  frame "Take LDA data" {
                    n517 = global read "Meas_global.vi" "Synchronise with LDA"() -> (w912:bool)
                    n518 = global read "Meas_global.vi" "Ch & spans"() -> (w915:T26[])
                    n519 = global read "LDA_meas_global_1.vi" "Probe Configuration"() -> (w905:string)
                    n520 = Array Size(array=w915) -> (size(s)=w914:i32)
                    n521 = Greater Than 0?(x=w914) -> (x > 0?=w913:bool)
                    n522 = Compound Arithmetic op=AND(w912, w907, w913) -> (w911:bool)
                    n523 = Select(t="Synchronised with LDA", s=w911, f="") -> (s? t:f=w908:string)
                    n524 = Build Array(w905, w908) -> (w906:string[])
                  }
                }
                n525 = Compound Arithmetic op=AND(w899, w902) -> (w896:bool)
                n526 = Select(t="Continuous Time Trace", s=w896, f="") -> (s? t:f=w894:string)
                n527 = Build Array (concatenate)(w895, w894) -> (w893:string[])
                n528 = Build Array(w893) -> (w892:string[][])
                n529 = Transpose 2D Array(2D array=w892) -> (transposed array=w891:string[][])
                n530 = local write "BSA Diagnostic info"(w891) -> ()
              }
            }
          }
        }
      }
      frame #18 {
        n531 = local read "File"() -> (w933:T9)
        n532 = Equal?(x=Setup."Run Program" ("setup"), y=w934) -> (x = y?=w931:bool)
        n533 = Not Equal?(x=w933, y=Save_Data."Save No Data" ("File")) -> (x != y?=w932:bool)
        n534 = global read "Meas_global.vi" "Repeat Measurement?"() -> (w916:bool)
        n535 = Compound Arithmetic op=AND(invert w916, w931, w932) -> (w930:bool)
        n536 = Get Date/Time In Seconds() -> (seconds since 1Jan1904=w927:timestamp)
        n537 = To Double Precision Float(number=w927) -> (double precision float=w919:dbl)
        n538 = local read "Setup filename"() -> (w928:string)
        n539 = global read "Trav_pos_global.vi" "Meas Setup Number"() -> (w925:i32)
        n540 = global read "Meas_global.vi" "Board type"() -> (w923:T13)
        n541 = Greater Than 0?(x=w925) -> (x > 0?=w921:bool)
        n542 = Equal?(x=w923, y=Board_Types."Simulate" ("Board type")) -> (x = y?=w922:bool)
        n543 = And(x=w921, y=w922) -> (x .and. y?=w920:bool)
        n544 = case shown="True" w920 {
          tunnel: w919 -> [_ w938]
          tunnel: [w935 w936] -> w918
          tunnel: w917 -> [w935 _]
          frame False {
          }
          frame True {
            n545 = global read "Trav_pos_global.vi" "Current Row"() -> (w941:T17)
            n546 = Unbundle By Name(w941) -> ("Averaging time (min)"=w939:dbl)
            n547 = Multiply(x=60.0 ("y"), y=w939) -> (x*y=w937:dbl)
            n548 = Subtract(x=w938, y=w937) -> (x-y=w936:dbl)
          }
        }
        n549 = case shown="True" w930 {
          tunnel: w933 -> [_ _]
          tunnel: w919 -> [w944 w996]
          tunnel: w928 -> [w943 w995]
          tunnel: w918 -> [w942 w994]
          frame True {
            n550 = stacked-sequence {
              seq-local: [_ w948 _ _ _] -> [_ _ w954 _ _]
              seq-local: [_ _ _ w967 _] -> [_ _ _ _ w987]
              tunnel: w944 -> [w947 _ _ _ _]
              tunnel: w943 -> [w946 _ _ _ _]
              tunnel: w942 -> [w945 _ _ _ _]
              frame #0 {
                n551 = call "Write_Results_file.vi"("Experiment start time"=w945, "Experiment End time"=w947, "Setup filename"=w946) -> ()  [unwired: 4 out]
              }
              frame #1 {
                n552 = global read "Meas_global.vi" "Second Graph"() -> (w952:T3)
                n553 = global read "Meas_global.vi" "First Graph"() -> (w953:T3)
                n554 = Unbundle By Name(w952) -> ("Save graph"=w950:u16)
                n555 = Unbundle By Name(w953) -> ("Save graph"=w951:u16)
                n556 = Add(x=w951, y=w950) -> (x+y=w949:u16)
                n557 = Not Equal To 0?(x=w949) -> (x != 0?=w948:bool)
              }
              frame #2 {
                n558 = case shown="True" w954 {
                  frame False {
                  }
                  frame True {
                    n559 = stacked-sequence {
                      tunnel: "Show Smoth" -> [w958 w959]
                      frame #0 {
                        n560 = local read "First plot"() -> (w957:cluster{"Xo":dbl, "Delta X":dbl, dbl[]}[])
                        n561 = local read "2nd plot"() -> (w956:cluster{"Xo":dbl, "Delta X":dbl, dbl[]}[])
                        n562 = call "Save_plot_routine.vi"("Show Smooth"=w958, "First Plot data"=w957, "Second Plot data"=w956) -> ()  [unwired: 1 in, 3 out]
                      }
                      frame #1 {
                        n563 = case shown="True" w959 {
                          frame False {
                          }
                          frame True {
                            n564 = Open VI Reference(vi path="Measurement.vi") -> (vi reference=w965:refnum<vi>, error out=w961:errorcluster)  [unwired: 1 in, 4 out]
                            n565 = local write "Show Smoth"(FALSE ("Show Smoth")) -> ()
                            n566 = property class="VI"(reference=w965, error in=w961, "Front Panel Window:Is Frontmost"=TRUE) -> (reference out=w963:refnum<vi>, error out=w962:errorcluster)
                            n567 = Close Reference(reference=w963, error in (no error)=w962) -> ()  [unwired: 1 out]
                          }
                        }
                      }
                    }
                  }
                }
              }
              frame #3 {
                w972 = FALSE  # Empty list
                n568 = global read "Meas_global.vi" "Raw data file"() -> (w971:path)
                n569 = global read "Trav_pos_global.vi" "Top level setup filename"() -> (w969:path)
                n570 = global read "Meas_global.vi" "Start Time of experiment"() -> (w968:dbl)
                n571 = Strip Path(path=w971) -> (stripped path=w967:path)  [unwired: 1 out]
                n572 = Empty String/Path?(string/path=w969) -> (empty?=w970:bool)
                n573 = case shown="False" w970 {
                  tunnel: w969 -> [w986 _]
                  tunnel: w967 -> [w984 _]
                  tunnel: w968 -> [w982 _]
                  frame False {
                    n574 = call "Sec_to_date_filename.vi"("seconds"=w982) -> ("Day"=w981:string, "Time"=w980:string)  [unwired: 2 out]
                    n575 = Format Into String(format string="Cmd_%s_%s.xls", w981, w980) -> (resulting string=w978:string)  [unwired: 2 in, 1 out]
                    n576 = call "Fast_string_Replace.vi"("Replace match with:"="-", "Input String"=w978, "regular expression"=":") -> ("Output String"=w975:string)  [unwired: 2 out]
                    n577 = call "Fast_string_Replace.vi"("Replace match with:"="", "Input String"=w975, "regular expression"=" ") -> ("Output String"=w973:string)  [unwired: 2 out]
                    n578 = Build Path(base path=w984, name or relative path=w973) -> (appended path=w983:path)
                    n579 = Copy(10:w983, 11:w986) -> ()  [unwired: 1 in, 5 out]
                  }
                  frame True {
                  }
                }
                n580 = call "Remember_RD_Folders.vi"("Empty list"=w972, "Folders to Remember"=w967) -> ()  [unwired: 1 out]
              }
              frame #4 {
                n581 = global read "Meas_global.vi" "LDA data"() -> (w988:enum16{"No LDA data", "Take LDA data"})
                n582 = case shown="\"Take LDA data\"" w988 {
                  tunnel: w987 -> [_ w992]
                  frame "No LDA data" {
                  }
                  frame "Take LDA data" {
                    w990 = "LDA_Probe_Orientation.txt" ("name or relative path")
                    n583 = call "Setup_Filepath.vi"("Setup File Type"=Setup_Filetype."General", "Filename in"=w990) -> ("Filename Out"=w989:path)  [unwired: 1 out]
                    n584 = Build Path(base path=w992, name or relative path=w990) -> (appended path=w993:path)
                    n585 = Copy(10:w993, 11:w989) -> ()  [unwired: 1 in, 5 out]
                  }
                }
              }
            }
          }
          frame False {
            n586 = global read "Meas_global.vi" "Raw data option"() -> (w997:enum16{"Save raw data", "Raw data not saved"})
            n587 = case shown="\"Save raw data\"" w997 {
              tunnel: w994 -> [w1000 _]
              tunnel: w996 -> [w999 _]
              tunnel: w995 -> [w998 _]
              frame "Save raw data" {
                n588 = stacked-sequence {
                  tunnel: w1000 -> [_ w1009]
                  tunnel: w999 -> [_ w1008]
                  tunnel: w998 -> [_ w1006]
                  frame #0 {
                    n589 = global read "Meas_global.vi" "Current Block No"() -> (w1001:i32)
                    n590 = global write "Meas_global.vi" "Requested No of blocks"(w1001) -> ()
                  }
                  frame #1 {
                    n591 = call "Create_Raw_data_file.vi"("No of averages"=1, "End time"=w1008, "Start time"=w1009, "Setup filename"=w1006) -> ("Values"=w1004:string[][], "Column headers"=w1005:string[])  [unwired: 2 out]
                    n592 = Index Array(array=w1004, index (row)=0) -> (element=w1002:string[])  [unwired: 1 in]
                    n593 = global write "Dynamic_call_global.ph.vi" "Plug in values"(w1002) -> ()
                    n594 = global write "Dynamic_call_global.ph.vi" "Plug in titles"(w1005) -> ()
                  }
                }
              }
              frame "Raw data not saved" {
              }
            }
          }
        }
      }
      frame #19 {
        n595 = stacked-sequence {
          seq-local: [w1016 _] -> [_ w1025]
          seq-local: [w1012 _] -> [_ w1024]
          tunnel: w1010 -> [w1023 _]
          frame #0 {
            n596 = global read "Meas_global.vi" "Raw data file"() -> (w1014:path)
            n597 = global read "Meas_global.vi" "Raw data option"() -> (w1022:enum16{"Save raw data", "Raw data not saved"})
            n598 = Equal?(x=Setup."Run Program" ("setup"), y=w1023) -> (x = y?=w1018:bool)
            n599 = Strip Path(path=w1014) -> (stripped path=w1013:path)  [unwired: 1 out]
            n600 = Equal?(x=w1022, y=enum16{"Save raw data", "Raw data not saved"}."Save raw data" ("Raw data option")) -> (x = y?=w1017:bool)
            n601 = Build Path(base path=w1013, name or relative path="VI_History.xls") -> (appended path=w1012:path)
            n602 = call "Does_file_exist_(simple).vi"("Pathname"=w1012) -> ("exists?"=w1020:bool)
            n603 = Not(x=w1020) -> (.not. x?=w1019:bool)
            n604 = Compound Arithmetic op=AND(w1019, w1018, w1017) -> (w1016:bool)
          }
          frame #1 {
            n605 = case shown="True" w1025 {
              tunnel: w1024 -> [_ w1032]
              frame False {
              }
              frame True {
                w1026 = FALSE  # Lock File
                n606 = global read "Meas_global.vi" "Prog's last revision date"() -> (w1029:u32)
                n607 = Get Date/Time String(date format (0)=enum16{"short", "long", "abbreviated"}."abbreviated", seconds (now)=w1029) -> (date string=w1028:string)  [unwired: 2 out]
                n608 = call "Characters_to_string.vi"("Characters to write"=w1028, "Label for characters"="Prog's last revision date") -> ("Output string"=w1034:string)
                n609 = call "Date_and_Time_to_string.vi"() -> ("Date and time (spreadsheet)"=w1035:string)
                n610 = call "Get_mod_dates.vi"() -> ("error out"=w1033:errorcluster, "Output string"=w1027:string)  [unwired: 1 in, 3 out]
                n611 = call "EnFlo_Error_Handler.vi"("error in (no error)"=w1033) -> ()  [unwired: 2 in, 3 out]
                n612 = Concatenate Strings(w1035, w1034, w1027) -> (w1031:string)
                n613 = call "Write_Characters_To_File.vi"("file path (dialog if empty)"=w1032, "character string"=w1031, "Lock File"=w1026) -> ()  [unwired: 2 in, 4 out]
              }
            }
          }
        }
      }
      frame #20 {
        w1039 = FALSE ("Remote control")
        n614 = local read "Correlate?"() -> (w1041:T6)
        n615 = case shown="\"Run Program\"" w1038 {
          tunnel: w1038 -> [w1045 _ _ _]
          tunnel: [w1045 w1062 w1063 w1064] -> w1037
          frame "Run Program" {
            n616 = global read "Meas_global.vi" "Velocity Cluster Array"() -> (w1044:T27[])
            n617 = Array Size(array=w1044) -> (size(s)=w1043:i32)
            n618 = Decrement(x=w1043) -> (x-1=w1042:i32)
            n619 = while {
              tunnel: w1044 -> [w1060] mode=indexing
              tunnel: w1042 -> [w1051]
              i -> [w1052]
              stop <- w1049 continue-if-true
              w1057 = "Pitot ("
              n620 = Unbundle By Name(w1060) -> ("U"=w1046:dbl, "Name"=w1056:string)
              n621 = String Length(string=w1057) -> (length=w1059:i32)
              n622 = String Subset(string=w1056, length (rest)=w1059) -> (substring=w1058:string)  [unwired: 1 out]
              n623 = Equal?(x=w1058, y=w1057) -> (x = y?=w1053:bool)
              n624 = call "Match_Pat_Case_In.vi"("String to match"="ref", "String"=w1056) -> ("offset past match"=w1054:i32)  [unwired: 1 in, 3 out]
              n625 = Greater Or Equal To 0?(x=w1054) -> (x >= 0?=w1048:bool)
              n626 = Less?(x=w1052, y=w1051) -> (x < y?=w1050:bool)
              n627 = And(x=w1048, y=w1053) -> (x .and. y?=w1047:bool)
              n628 = case shown="True" w1047 {
                tunnel: w1046 -> [_ w1061]
                frame False {
                }
                frame True {
                  n629 = call "Log_Reference_Velocity.vi"("Measured Velocity"=w1061) -> ()  [unwired: 1 out]
                }
              }
              n630 = Compound Arithmetic op=AND(invert w1047, w1050) -> (w1049:bool)
            }
          }
          frame "Show Setup" {
            w1062 = Setup."Run Program"  # setup
          }
          frame "Save Current Setup" {
            w1063 = Setup."Run Program"  # setup
          }
          frame "Setup Front Panel" {
            w1064 = Setup."Run Program"  # setup
          }
        }
        n631 = case shown="\"Correlate without activating panel\"" w1041 {
          tunnel: [T6."Cross correlation off" T6."Correlate without activating panel" T6."Correlate without activating panel"] -> w1040
          frame "Cross correlation off" {
          }
          frame "Show correlation panel" {
          }
          frame "Correlate without activating panel" {
          }
        }
        n632 = local write "Correlate?"(w1040) -> ()
        n633 = global write "Meas_global.vi" "Remote control"(w1039) -> ()
        n634 = global write "Dynamic_call_global.ph.vi" "Acquisition Interlock"(w1039) -> ()
        n635 = call "Program_Active.vi"() -> ()  [unwired: 1 in]
        n636 = local write "setup"(w1037) -> ()
      }
      frame #21 {
        w1072 = FALSE  # Dialog Box (T)
        n637 = global read "Meas_global.vi" "Over/Under string"() -> (w1070:string)
        n638 = Empty String/Path?(string/path=w1070) -> (empty?=w1069:bool)
        n639 = Not(x=w1069) -> (.not. x?=w1068:bool)
        n640 = Bundle By Name(cluster=errorcluster {"status"=FALSE, "code"=0, "source"=""} ("error in (no error)"), "source"=w1070, "status"=w1068) -> (w1073:errorcluster)
        n641 = call "EnFlo_Error_Handler.vi"("error in (no error)"=w1073, "Error Type"="Signal Clipping", "Dialog Box (T)"=w1072) -> ()  [unwired: 3 out]
      }
      frame #22 {
        w1077 = string[] [] ("Per Block Plug Ins Extra")
        n642 = Empty String/Path?(string/path=w1081) -> (empty?=w1080:bool)
        n643 = global read "Dynamic_call_global.ph.vi" "Final Plug Ins"() -> (w1082:string[])
        n644 = case shown="True" w1080 {
          tunnel: w1081 -> [w1094 _]
          frame False {
            n645 = local read "Comments"() -> (w1093:string)
            n646 = call "Fast_string_Replace.vi"("Replace match with:"="", "Input String"=w1093, "regular expression"=w1094) -> ("Output String"=w1092:string)  [unwired: 2 out]
            n647 = local write "Comments"(w1092) -> ()
          }
          frame True {
          }
        }
        n648 = call "Plug_in_Directories.vi"() -> ("Final"=w1078:path)  [unwired: 3 out]
        n649 = for {
          tunnel: w1082 -> [w1097] mode=indexing
          tunnel: w1078 -> [w1096]
          w1100 = FALSE  # Dialog Box (T)
          n650 = Build Path(base path=w1096, name or relative path=w1097) -> (appended path=w1095:path)
          n651 = global read "Dynamic_call_global.ph.vi" "Plug in"() -> (w1105:refnum<vi>)
          n652 = Open VI Reference(type specifier VI Refnum (for type only)=w1105, vi path=w1095) -> (vi reference=w1104:refnum<vi>, error out=w1103:errorcluster)  [unwired: 2 in, 2 out]
          n653 = call-by-ref "?"(reference=w1104, error in=w1103) -> (reference out=w1101:refnum<vi>, error out=w1102:errorcluster)  [unwired: 6 in, 2 out]
          n654 = Close Reference(reference=w1101, error in (no error)=w1102) -> (error out=w1098:errorcluster)
          n655 = call "EnFlo_Error_Handler.vi"("error in (no error)"=w1098, "Error Type"="Running Final Plug In", "Dialog Box (T)"=w1100) -> ()  [unwired: 3 out]
        }
        n656 = global read "Meas_global.vi" "Repeat Measurement?"() -> (w1079:bool)
        n657 = case shown="False" w1079 {
          tunnel: w1076 -> [_ w1090]
          tunnel: [FALSE w1085] -> w1075
          frame False {
            n658 = global write "Trav_pos_global.vi" "Present Probe Positions"(T7 [] ("Present Probe Positions")) -> ()
          }
          frame True {
            n659 = global read "Meas_global.vi" "Post Process"() -> (w1088:T5)
            n660 = Equal To 0?(x=w1090) -> (x = 0?=w1086:bool)
            n661 = Equal?(x=w1088, y=Post_Process."Post Process Raw Data File" ("Post Process")) -> (x = y?=w1087:bool)
            n662 = And(x=w1087, y=w1086) -> (x .and. y?=w1085:bool)
          }
        }
        n663 = global write "Dynamic_call_global.ph.vi" "Per Block Plug Ins Extra"(w1077) -> ()
        n664 = global write "Dynamic_call_global.ph.vi" "Initial Plug Ins Extra"(w1077) -> ()
      }
      frame #23 {
        n665 = global read "Meas_global.vi" "Post Process"() -> (w1114:T5)
        n666 = local read "stop"() -> (w1120:bool)
        n667 = Equal?(x=w1115, y=Setup."Run Program" ("setup")) -> (x = y?=w1111:bool)
        n668 = Equal?(x=w1114, y=Post_Process."Take New Data" ("Post Process")) -> (x = y?=w1112:bool)
        n669 = And(x=w1111, y=w1112) -> (x .and. y?=w1110:bool)
        n670 = case shown="False" w1120 {
          tunnel: [Multi_Run_Status."Continue" ("Status Out") Multi_Run_Status."Terminate Run" ("Status Out")] -> w1118
          frame False {
          }
          frame True {
            n671 = local write "stop"(FALSE) -> ()
          }
        }
        n672 = global read "DataTranslation_global.vi" "Task ID"() -> (w1106:refnum<k24>)
        n673 = case shown="True" w1110 {
          tunnel: w1118 -> [w1127 w1130]
          tunnel: [w1127 w1132] -> w1117
          frame False {
          }
          frame True {
            n674 = local read "Raw data file"() -> (w1131:path)
            n675 = Path to Array of Strings(0:w1131) -> (2:w1133:string[])  [unwired: 1 out]
            n676 = Index Array(array=w1133, index=0 ("Index")) -> (element=w1129:string)
            n677 = Build Array(w1129) -> (w1128:string[])
            n678 = for {
              tunnel: w1128 -> [w1137] mode=indexing
              shift-right: [w1135] -> w1132
              shift-left: w1130 -> [w1136]
              n679 = call "Warn_on_low_HD_space.vi"("Status In"=w1136, "HD name"=w1137) -> ("Status Out"=w1135:T4)  [unwired: 6 out]
            }
          }
        }
        "Status Out" <- w1117
        n680 = Not A Number/Path/Refnum?(number/path/refnum=w1106) -> (NaN/Path/Refnum?=w1107:bool)
        n681 = case shown="False" w1107 {
          frame False {
            n682 = Open VI Reference(type specifier VI Refnum (for type only)=refnum<vi> refnum, vi path="Close_Data_Trans_Ref.vi") -> (vi reference=w1125:refnum<vi>, error out=w1121:errorcluster)  [unwired: 4 in]
            n683 = call-by-ref "?"(reference=w1125, error in=w1121) -> (reference out=w1123:refnum<vi>, error out=w1122:errorcluster)  [unwired: 1 out]
            n684 = Close Reference(reference=w1123, error in (no error)=w1122) -> ()  [unwired: 1 out]
          }
          frame True {
          }
        }
        n685 = global write "Trav_pos_global.vi" "Dummy Measurement?"(FALSE ("Dummy Measurement?")) -> ()
        n686 = global write "Plug_in_data_global.vi" "Server Channels to log"(string[] [] ("Server Channels to log")) -> ()
        n687 = global write "Meas_global.vi" "Extra Comments"("") -> ()
      }
    }
  }
